vi "Autonomous Independent.vi"() -> ()   [LabVIEW 2017]
doc: "This VI is called when autonomous begins, and will automatically be terminated when autonomous ends. You can carry out timed or sensor driven robot movement independently without needing to return to the caller."
uses:
  <vilib>/Rock Robotics/WPI/ThirdParty/Phoenix-LabVIEW/Motor Controller/Controls/CTRE_Phoenix_MotorControl_ControlMode.ctl
  <vilib>/Rock Robotics/WPI/Utilities/WPI_GetSetVariantRefNum.vi
  <vilib>/Rock Robotics/Network Tables/NT Read String.vi
  <vilib>/Rock Robotics/Network Tables/NT Write Numeric Array.vi
  <vilib>/Rock Robotics/WPI/ThirdParty/Phoenix-LabVIEW/Motor Controller/Get/CTRE_Phoenix_MotorController_GetClosedLoopData.vi
  <vilib>/addons/control/pid/pid.llb/PID (DBL).vi
  <vilib>/Rock Robotics/WPI/RobotDrive/WPI_RobotDriveArcadeDrive_Standard(NoSaturation).vi
  <vilib>/addons/control/pid/NI_PID_pid.lvlib
panel:
  in  "PID gains 3":T1={"proportional gain (Kc)"=0.17, "integral time (Ti, min)"=0.002, "derivative time (Td, min)"=0.0}
  in  "setpoint 3":dbl format="%.2f"
  out "Yaw 3":dbl
  out "Closed-loop Error RF 14":i32
  out "Closed-loop Error LR 14":i32
  out "Closed-loop Error RF 13":i32
  out "Closed-loop Error LR 13":i32
  in  "PID gains 2":T1={"proportional gain (Kc)"=0.17, "integral time (Ti, min)"=0.002, "derivative time (Td, min)"=0.0}
  in  "setpoint 2":dbl format="%.2f"
  out "Yaw 2":dbl
  out "Closed-loop Error RF 12":i32
  out "Closed-loop Error LR 12":i32
  out "Closed-loop Error RF 11":i32
  out "Closed-loop Error LR 11":i32
  in  "Acceleration":i32=2100
  in  "Cruise Velocity":i32=1500
  out "Closed-loop Error LR":i32
  out "Closed-loop Error RF":i32
  in  "Lt Target 1":dbl=36500.0
  # "Be sure to right-click and choose Data Operations>>Make Current Value default if you want to save the array values with the VI"
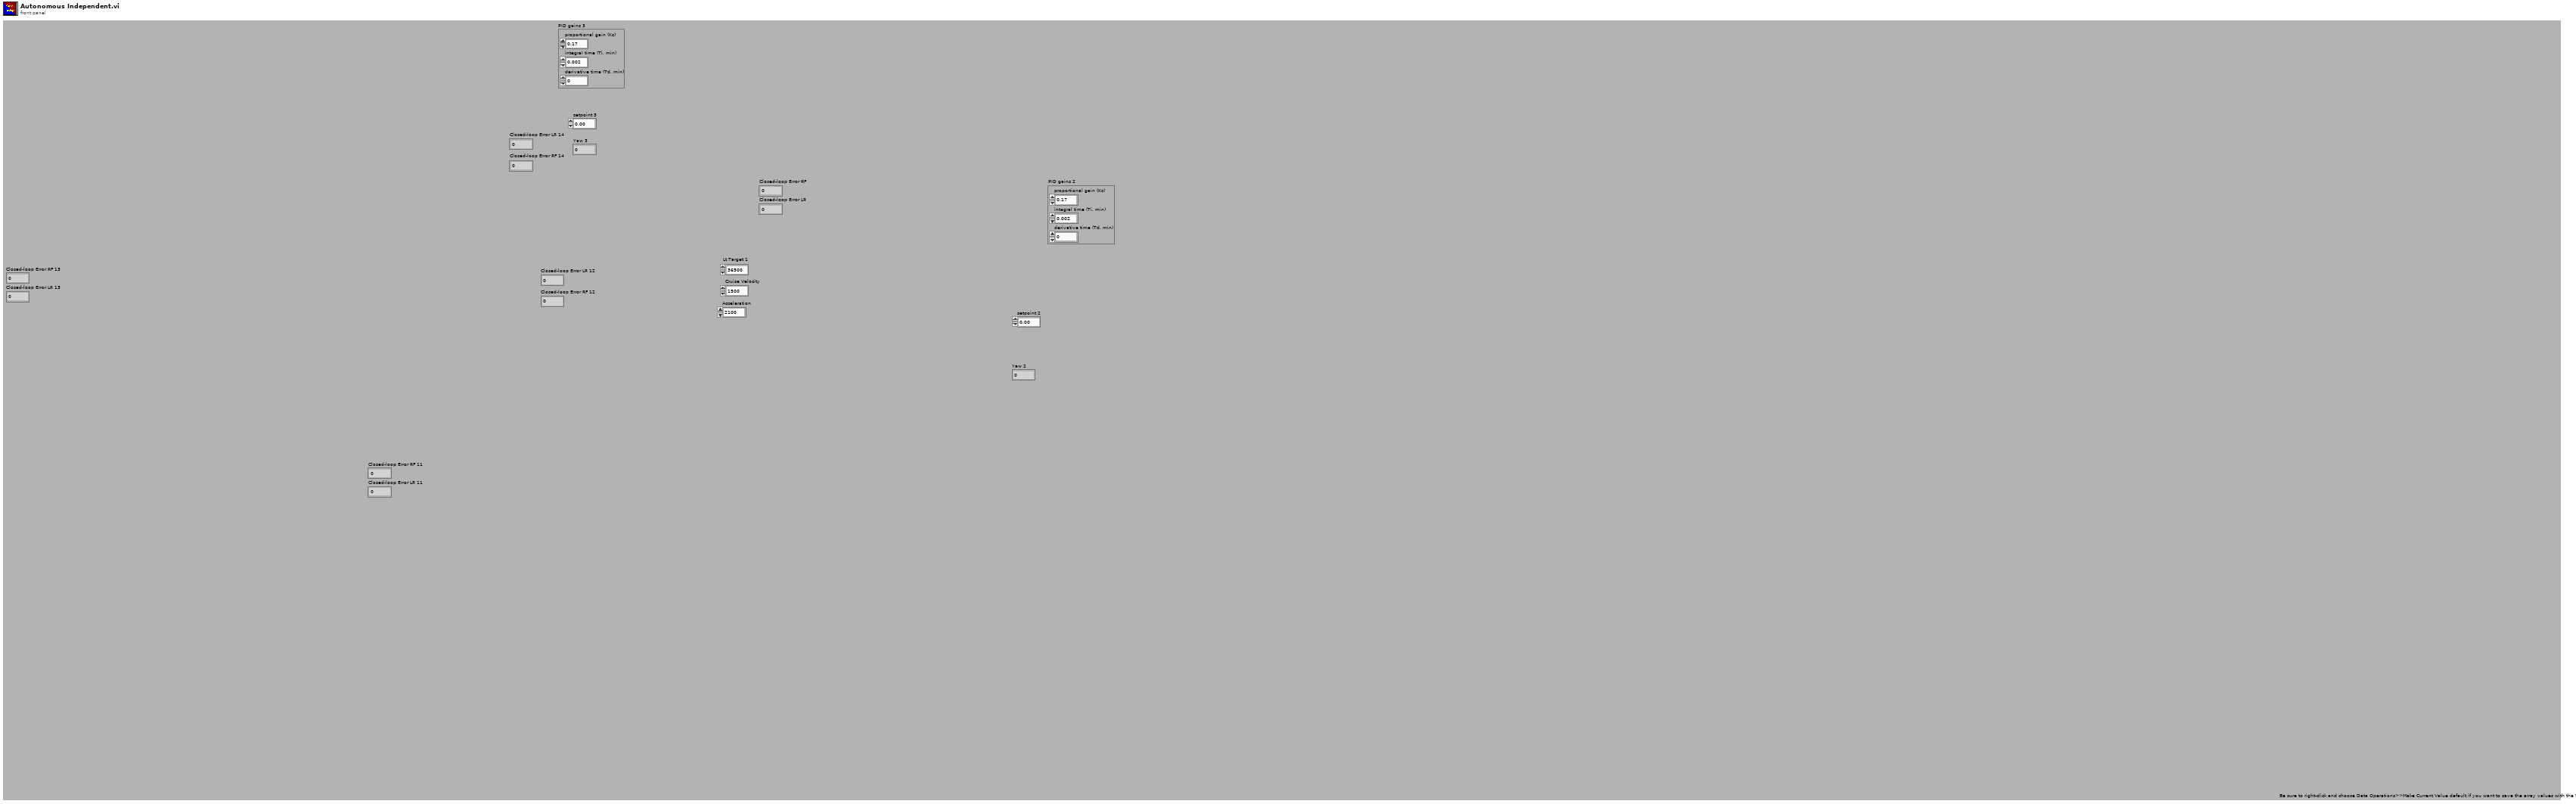
[diagram p1: front panel]
types:
  T1 = cluster{"proportional gain (Kc)":dbl, "integral time (Ti, min)":dbl, "derivative time (Td, min)":dbl}
  T2 = typedef "WPI_MotorControlDeviceRef.ctl" = cluster{"DeviceStatus":errorcluster, "Type":T3, "PWM":cluster{"PWM Channel":T4, "DeadBand":T5}, "CAN":cluster{"Device Number":u8, "SetOutput VI Ref":variant, "GetOutput VI Ref":variant, "Enable VI Ref":variant, "Disable VI Ref":variant, "Data":variant}, "Invert":bool, "DIO PWM":cluster{"PWM \"Enable\" Channel":T4, "DIOChannel":T6, "PWM Rate":dbl}}
  T3 = typedef "WPI_MotorControlType.ctl" = enum16{"PWM", "CAN", "DIO PWM"}
  T4 = typedef "FPGA_DIOPWMChannel.ctl" = enum8{"PWM 0", "PWM 1", "PWM 2", "PWM 3", "PWM 4", "PWM 5", "PWM 6", "PWM 7", "PWM 8", "PWM 9", "PWM MXP 0", "PWM MXP 1", "PWM MXP 2", "PWM MXP 3", "PWM MXP 4", "PWM MXP 5", "PWM MXP 6", "PWM MXP 7", "PWM MXP 8", "PWM MXP 9", "Invalid"}
  T5 = typedef "WPI_PWMDeadband.ctl" = cluster{"Name":string, "maxPositivePwm":i32, "minPositivePwm":i32, "centerPwm":i32, "maxNegativePwm":i32, "minNegativePwm":i32, "angularRange":u16}
  T6 = typedef "FPGA_DIOChannel.ctl" = enum8{"DIO 0", "DIO 1", "DIO 2", "DIO 3", "DIO 4", "DIO 5", "DIO 6", "DIO 7", "DIO 8", "DIO 9", "DIO MXP 0", "DIO MXP 1", "DIO MXP 2", "DIO MXP 3", "DIO MXP 4", "DIO MXP 5", "DIO MXP 6", "DIO MXP 7", "DIO MXP 8", "DIO MXP 9", "DIO MXP 10", "DIO MXP 11", "DIO MXP 12", "DIO MXP 13", "DIO MXP 14", "DIO MXP 15", "SPI Port CS1", "SPI Port CS2", "SPI Port CS3", "SPI Port MISO", "SPI Port MOSI", "Invalid"}
  T7 = typedef "WPI_JoystickDevRef.ctl" = cluster{"Device":T8}
  T8 = typedef "WPI_JoystickDeviceEnum.ctl" = enum16{"USB 0", "USB 1", "USB 2", "USB 3", "USB 4", "USB 5"}
  T9 = typedef "CTRE_Phoenix_MotorControl_ControlMode.ctl" = u16
  T10 = cluster{"Yaw":dbl, "Roll":dbl, "Pitch":dbl, "Heading":dbl, "Fused Heading":dbl}
  T11 = typedef "WPI_RobotDriveDevRef.ctl" = cluster{"DevStatus":errorcluster, "Motors[]":T2[], "Square Inputs":bool, "Max Output":dbl}
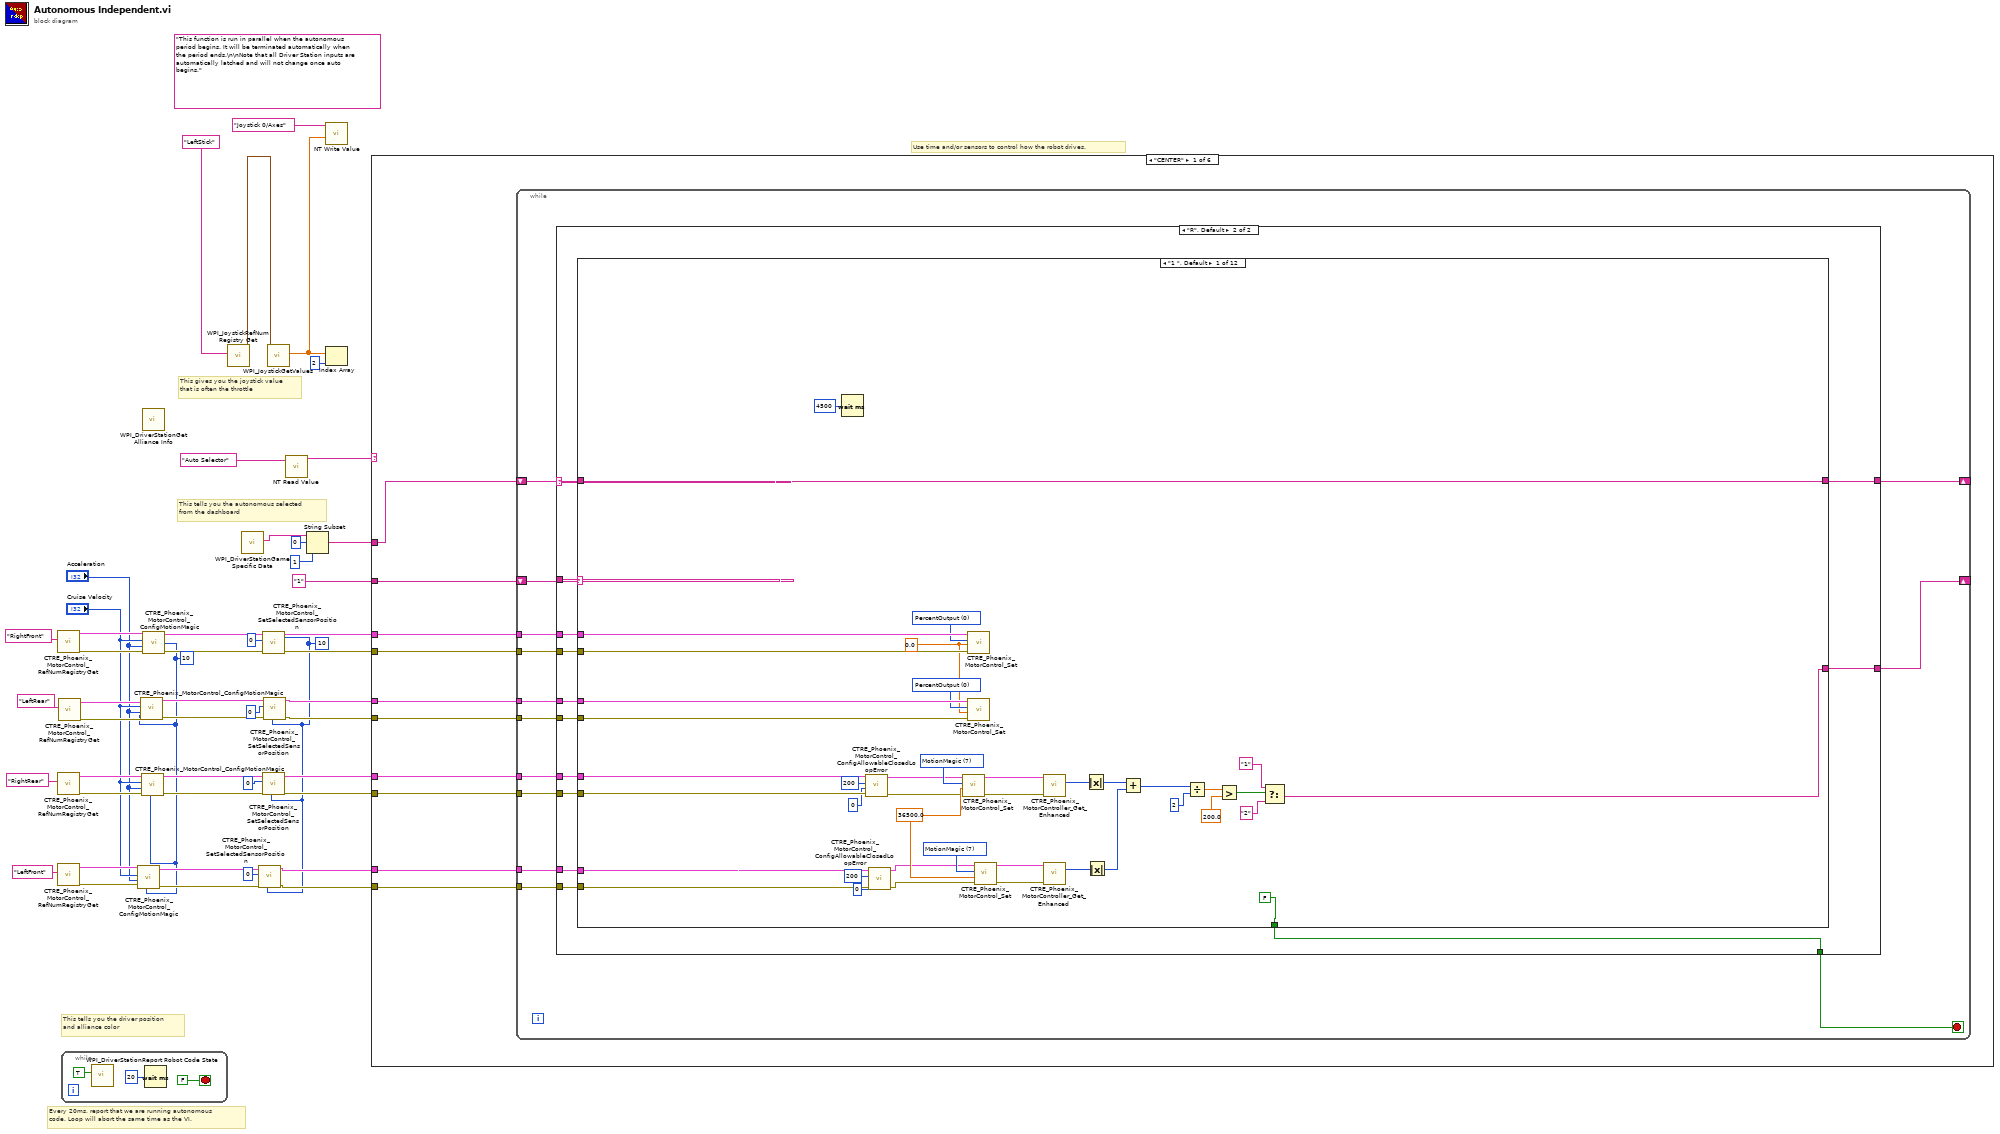
[diagram p0: block diagram]
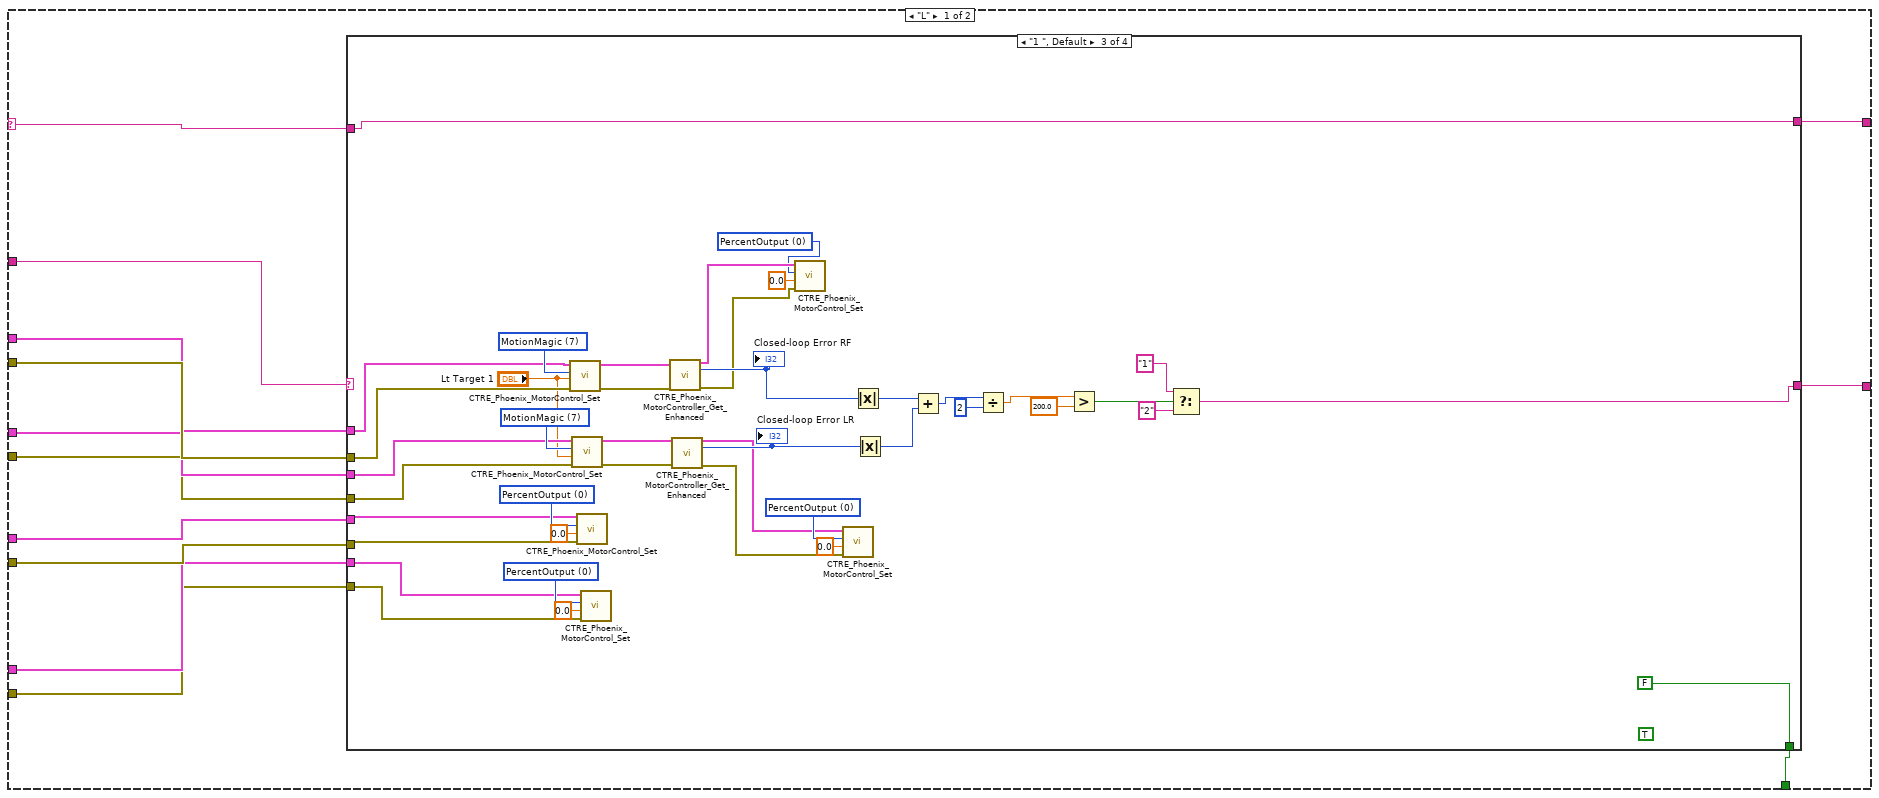
[diagram p2: hidden frame]
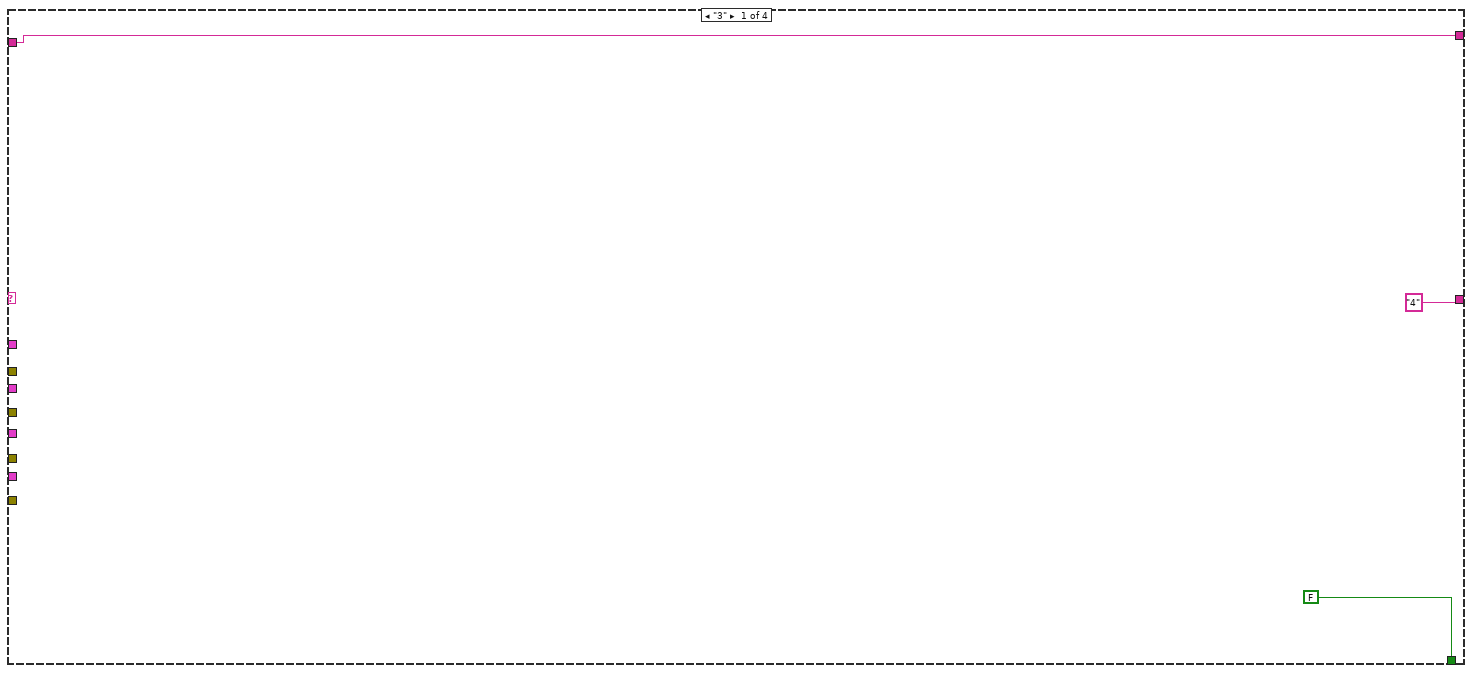
[diagram p3: hidden frame]
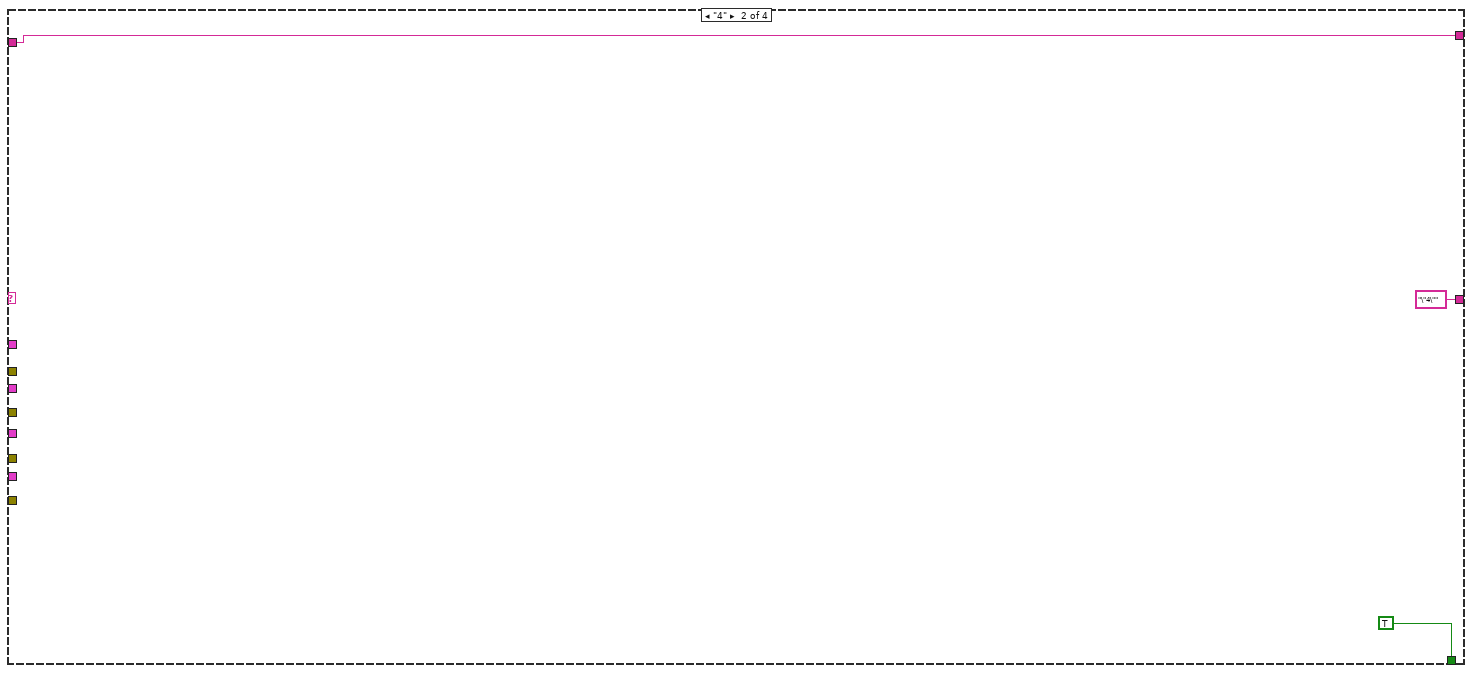
[diagram p4: hidden frame]
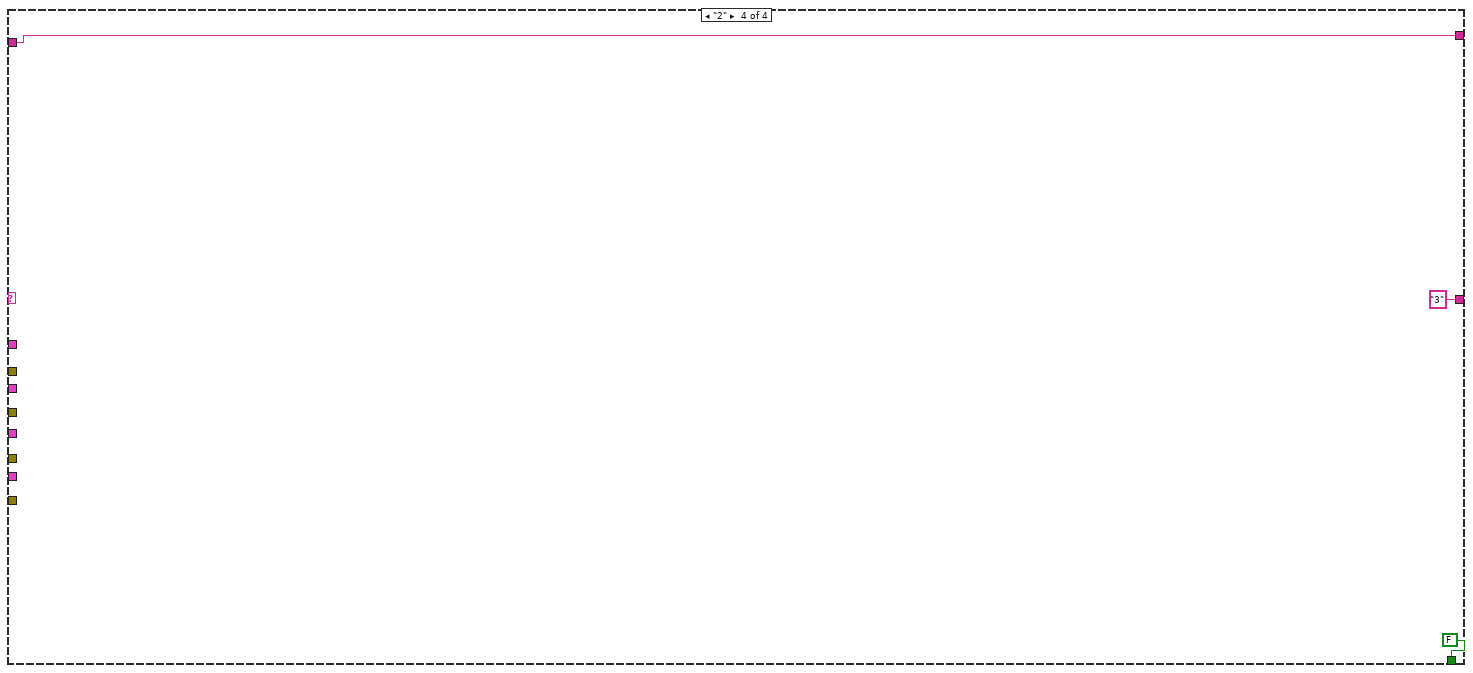
[diagram p5: hidden frame]
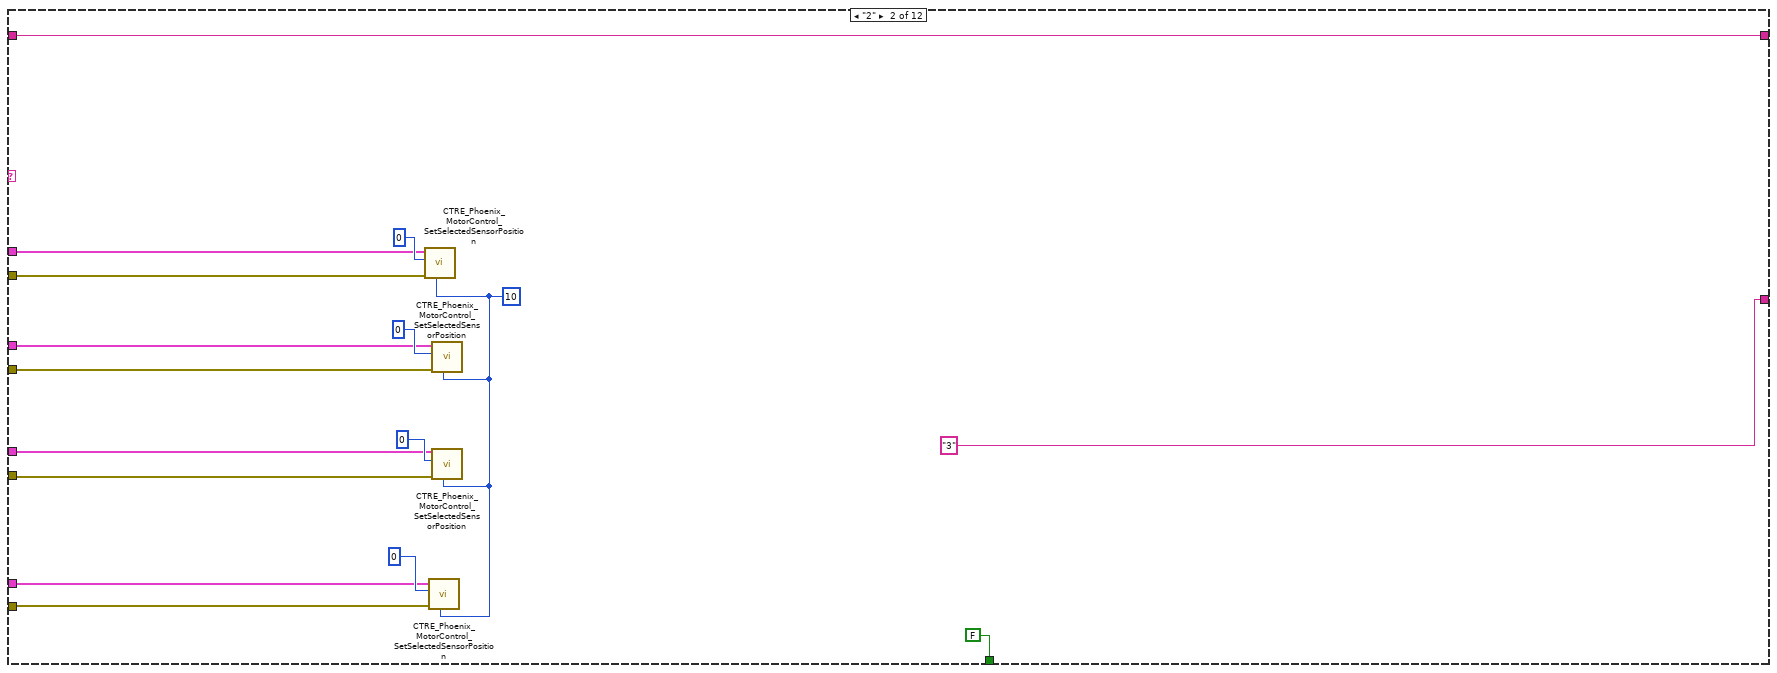
[diagram p6: hidden frame]
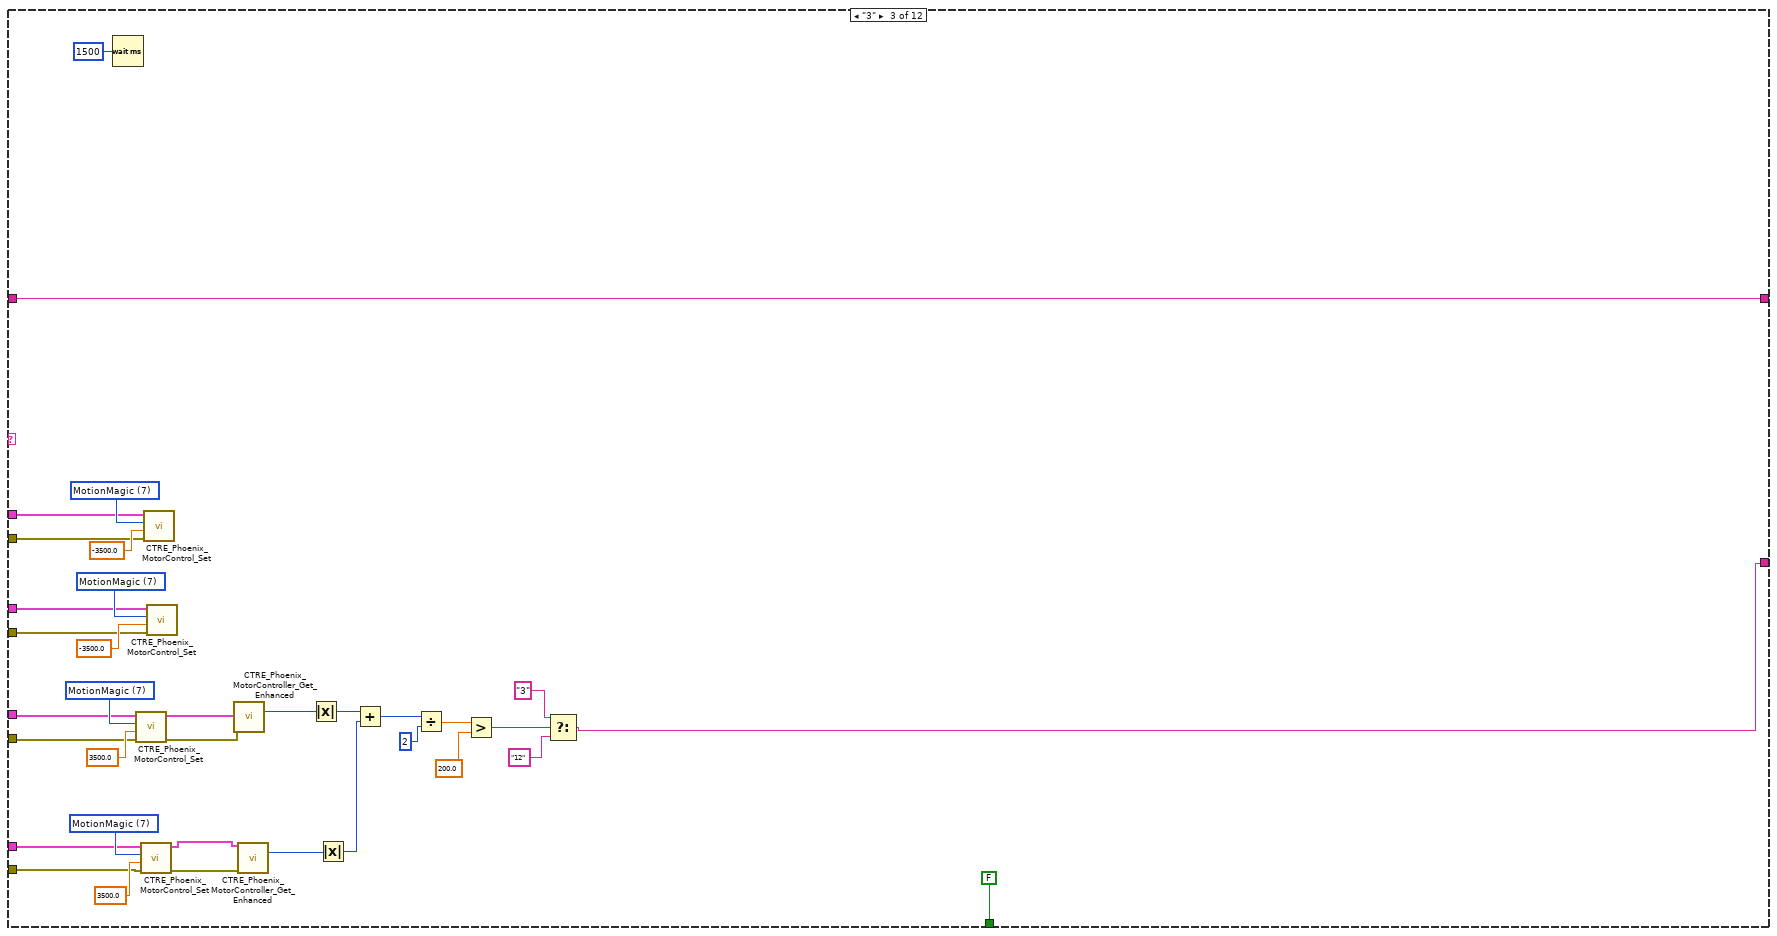
[diagram p7: hidden frame]
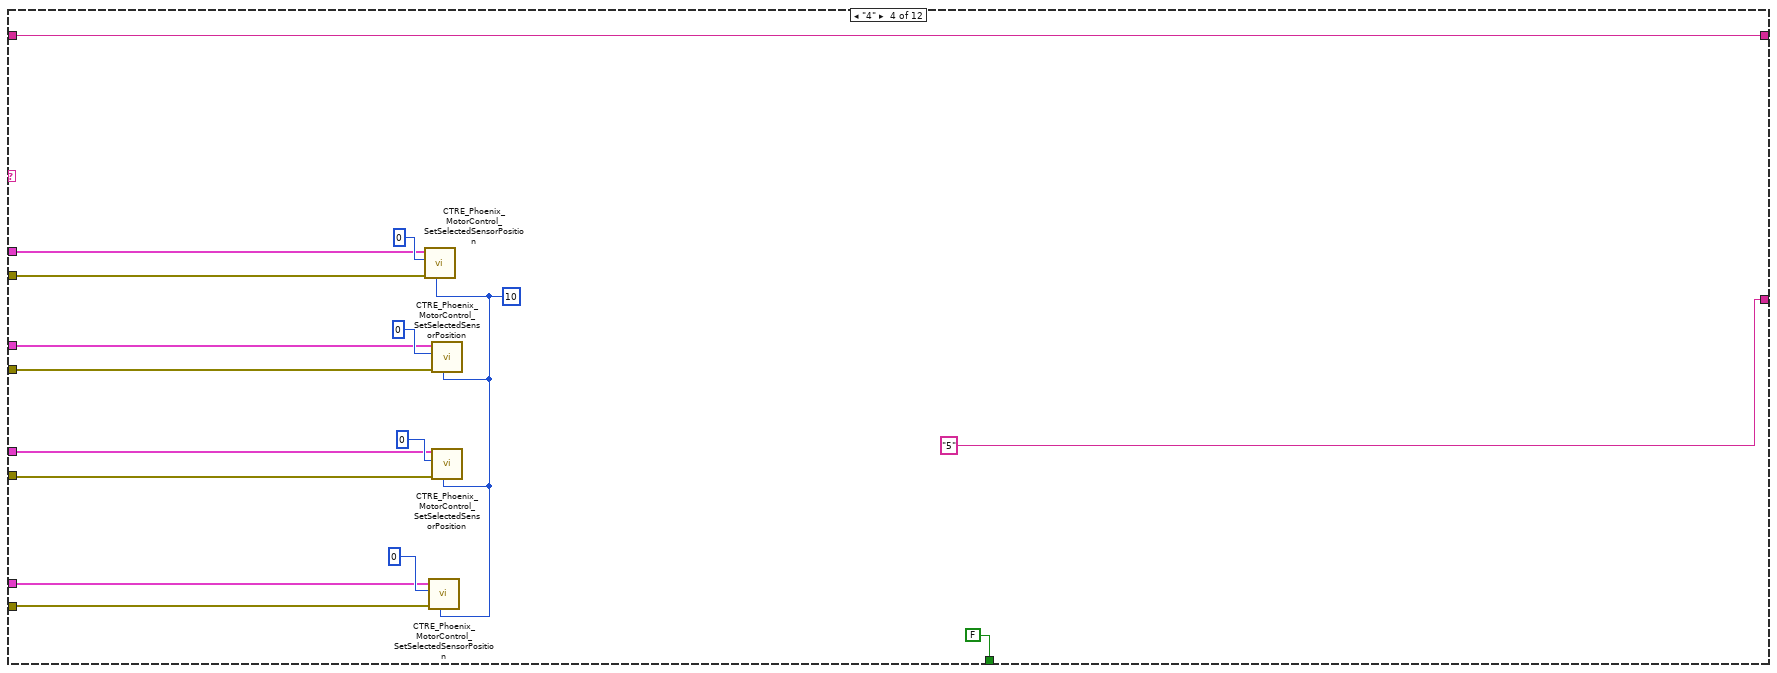
[diagram p8: hidden frame]
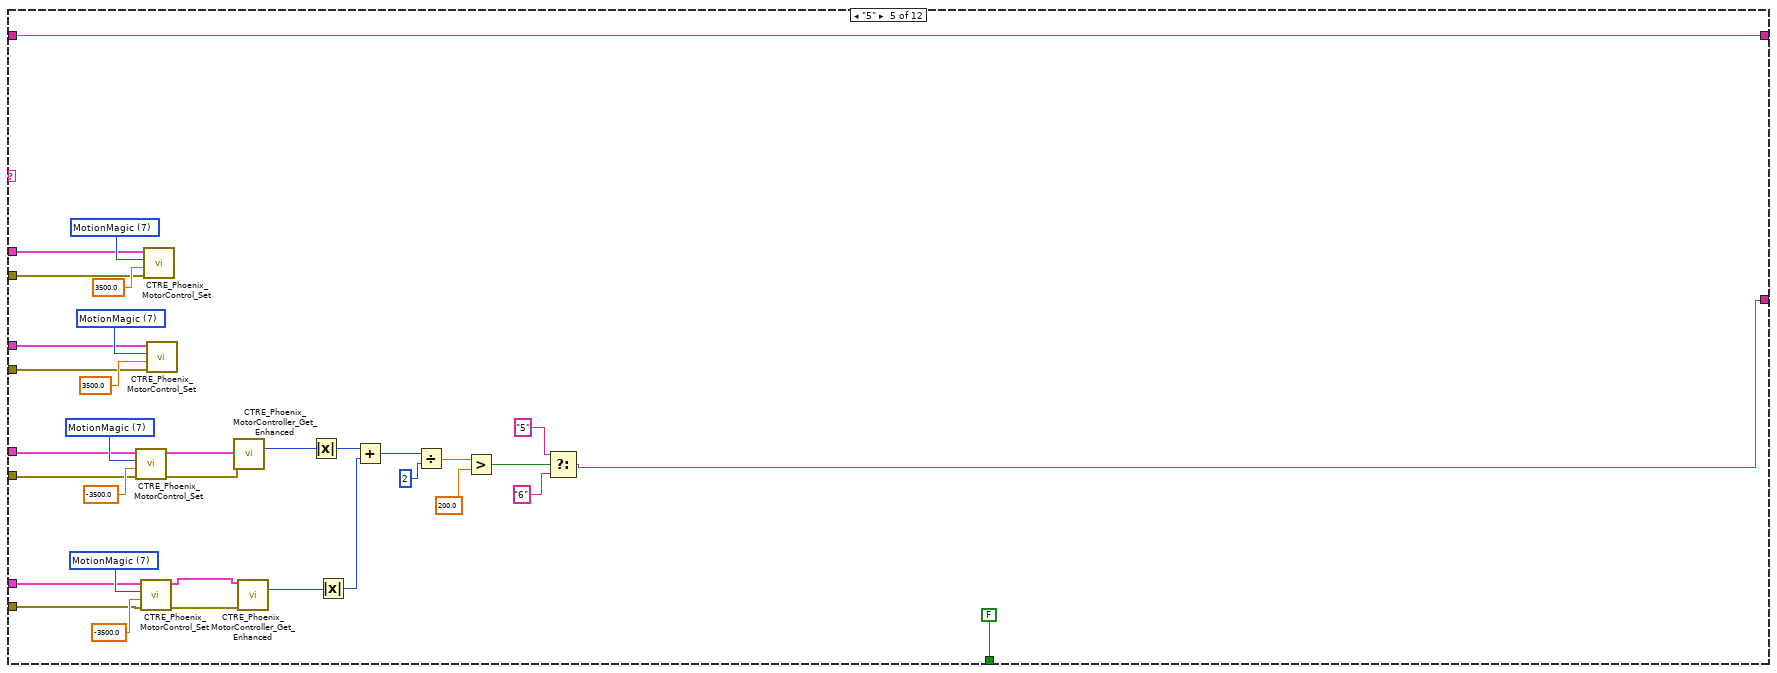
[diagram p9: hidden frame]
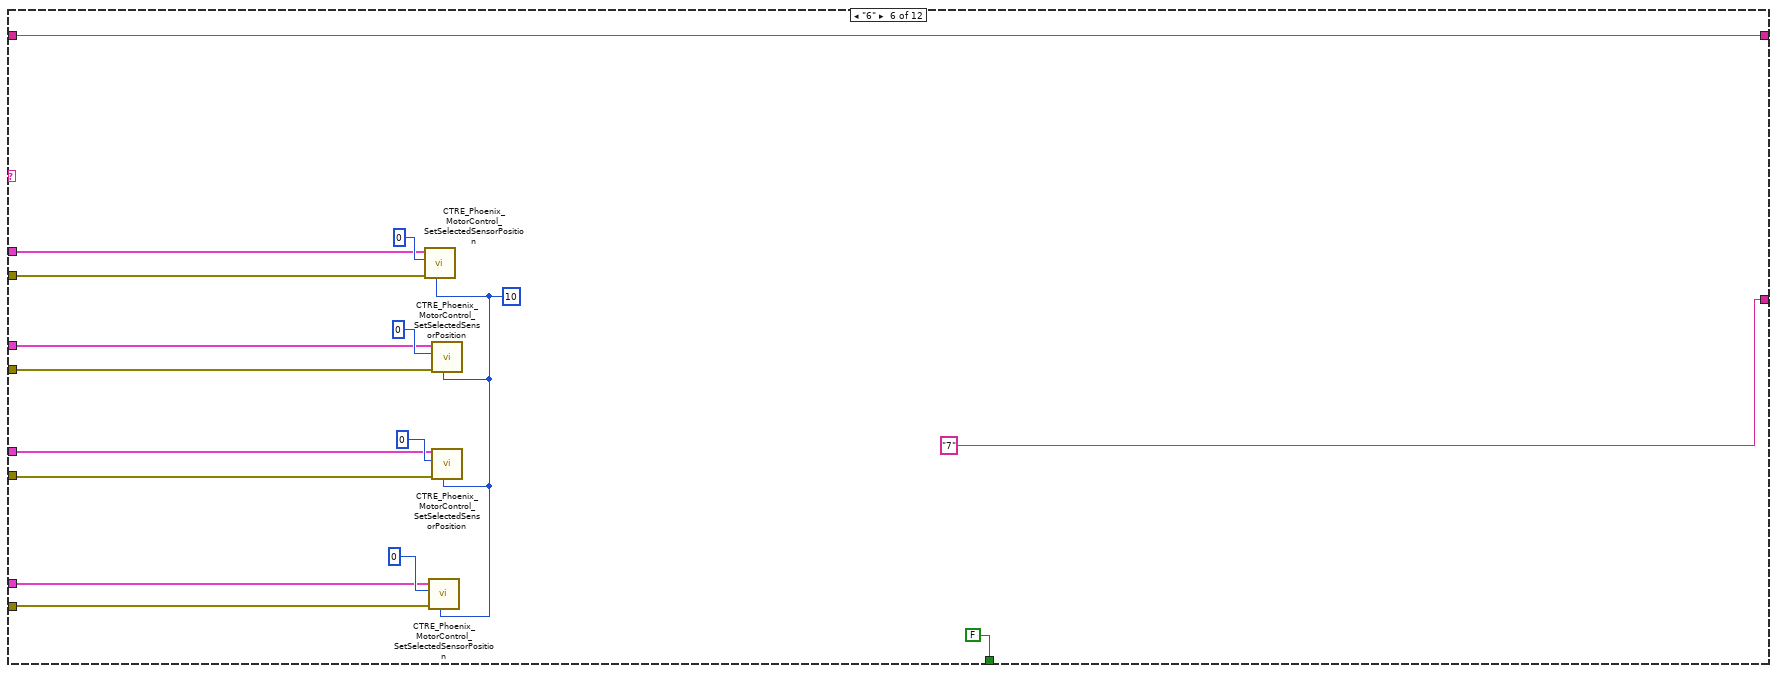
[diagram p10: hidden frame]
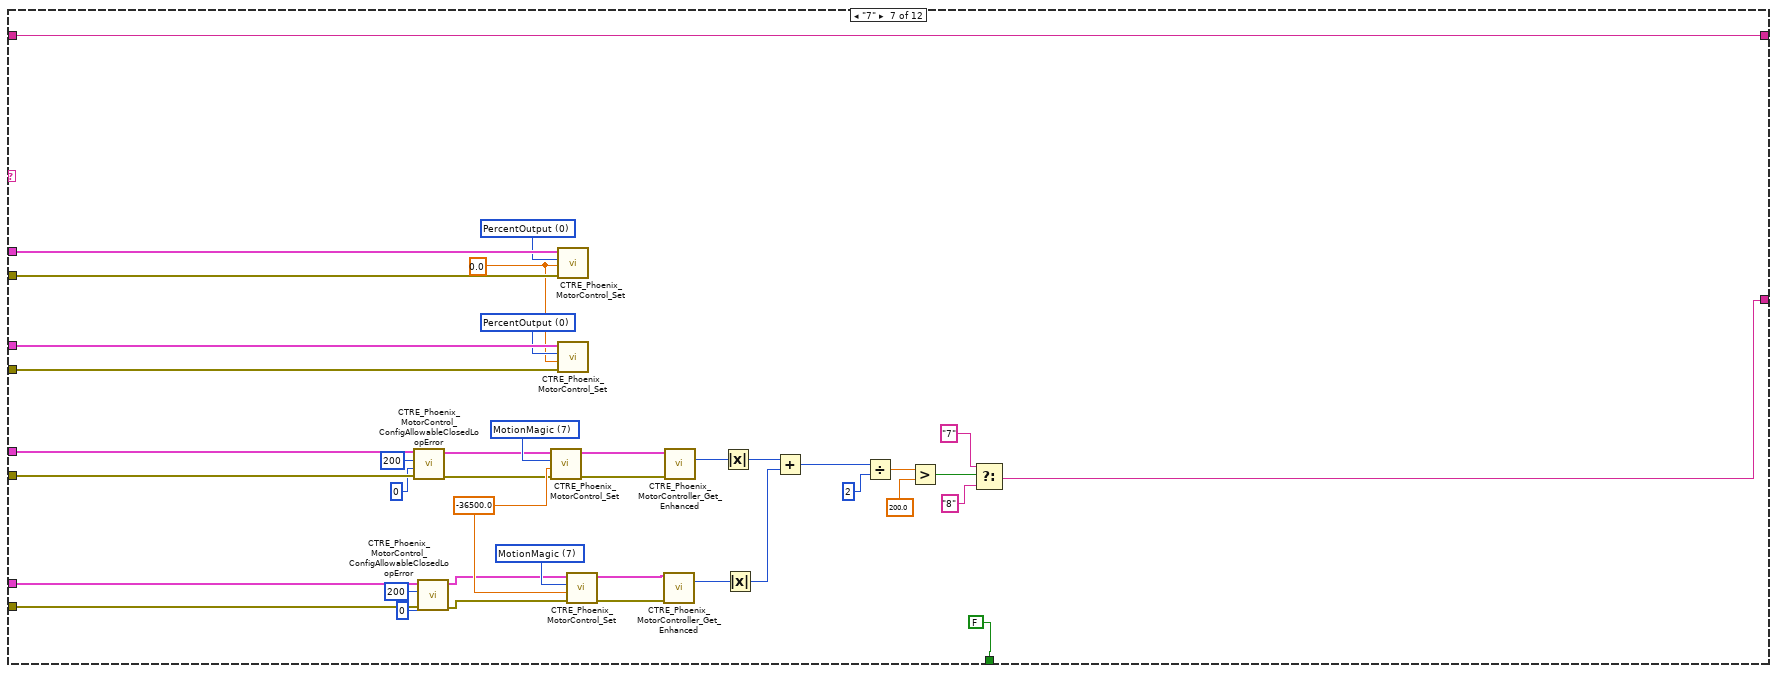
[diagram p11: hidden frame]
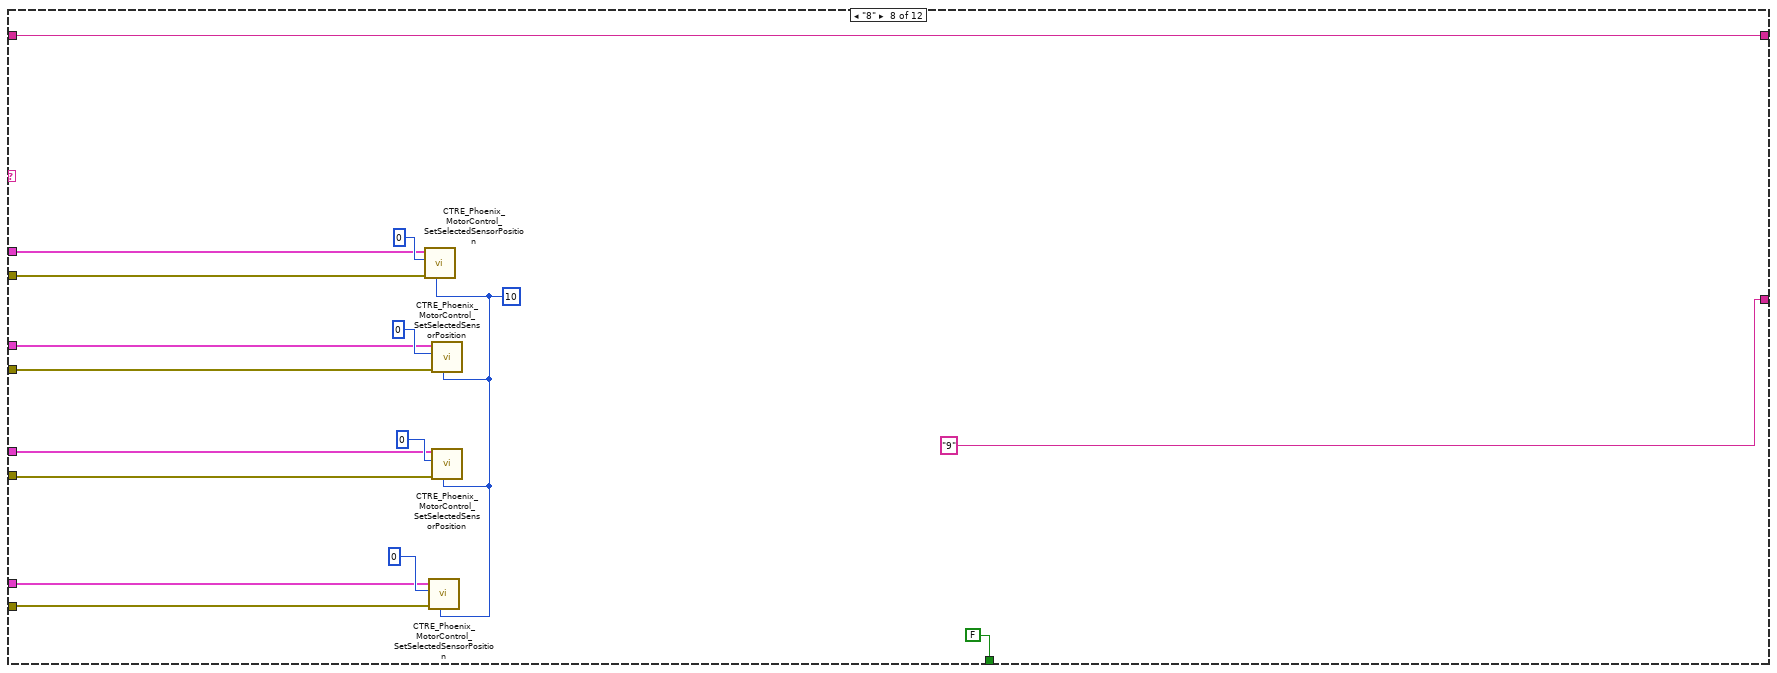
[diagram p12: hidden frame]
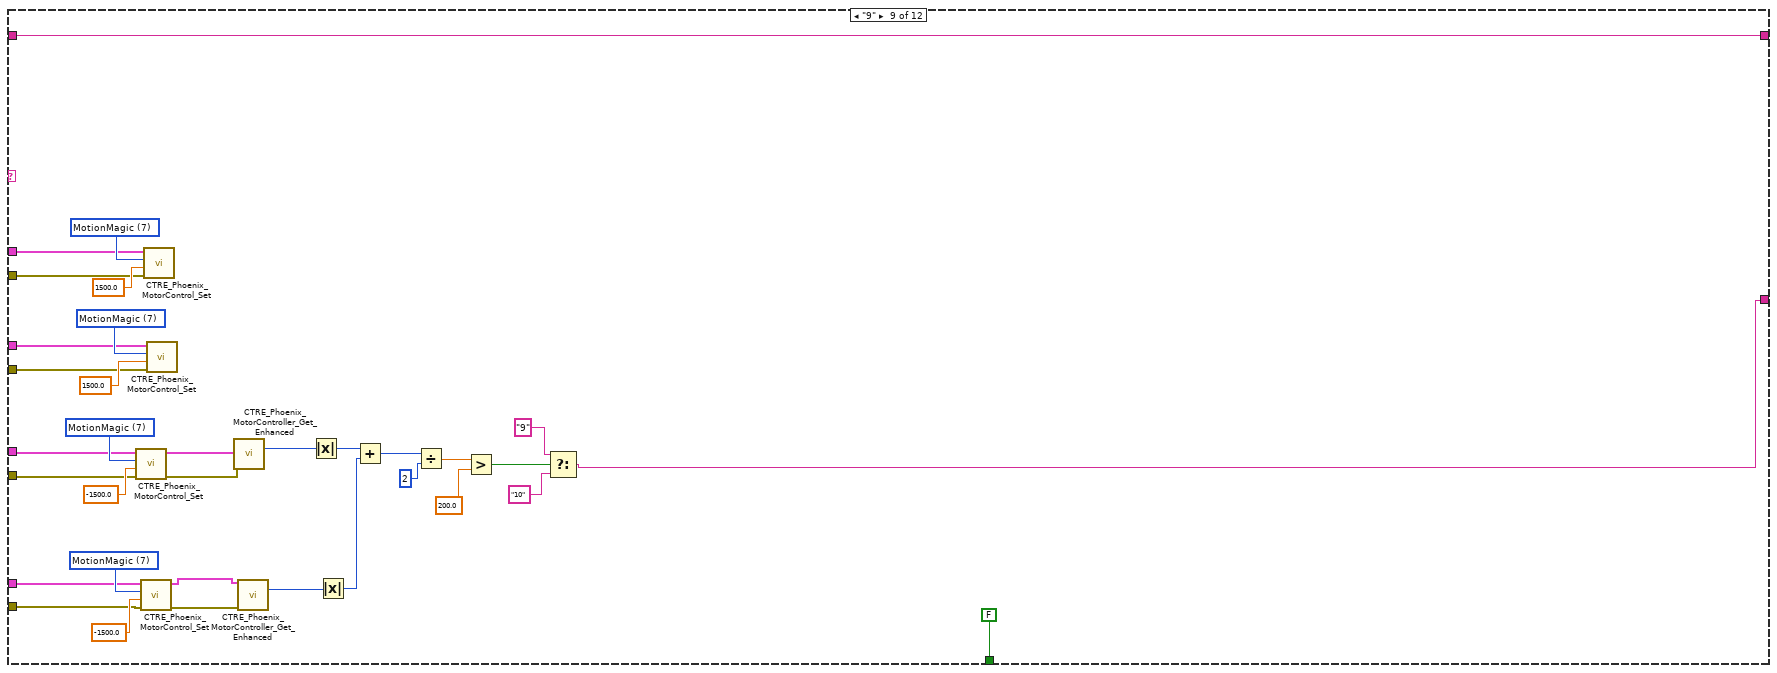
[diagram p13: hidden frame]
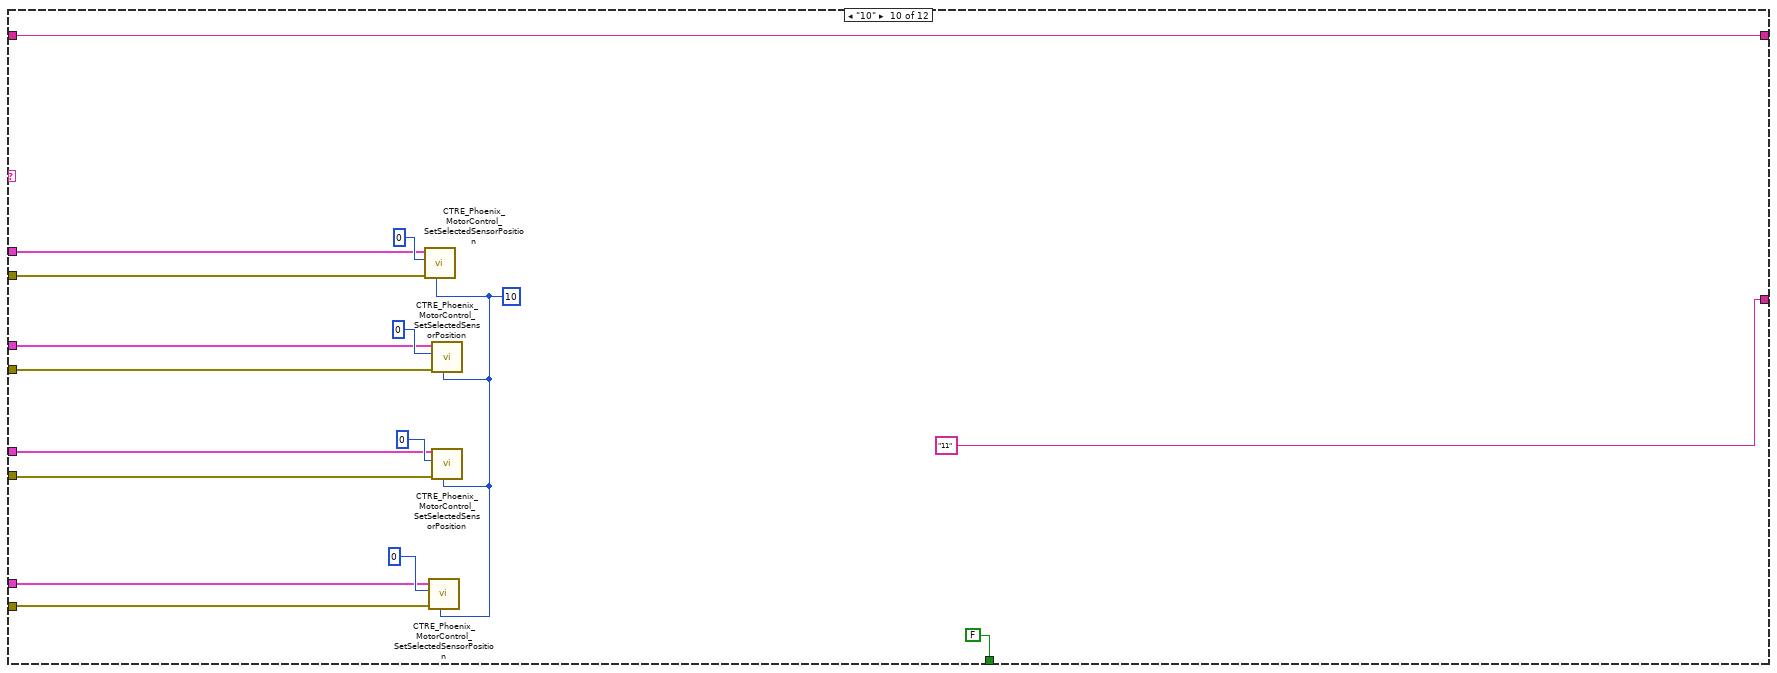
[diagram p14: hidden frame]
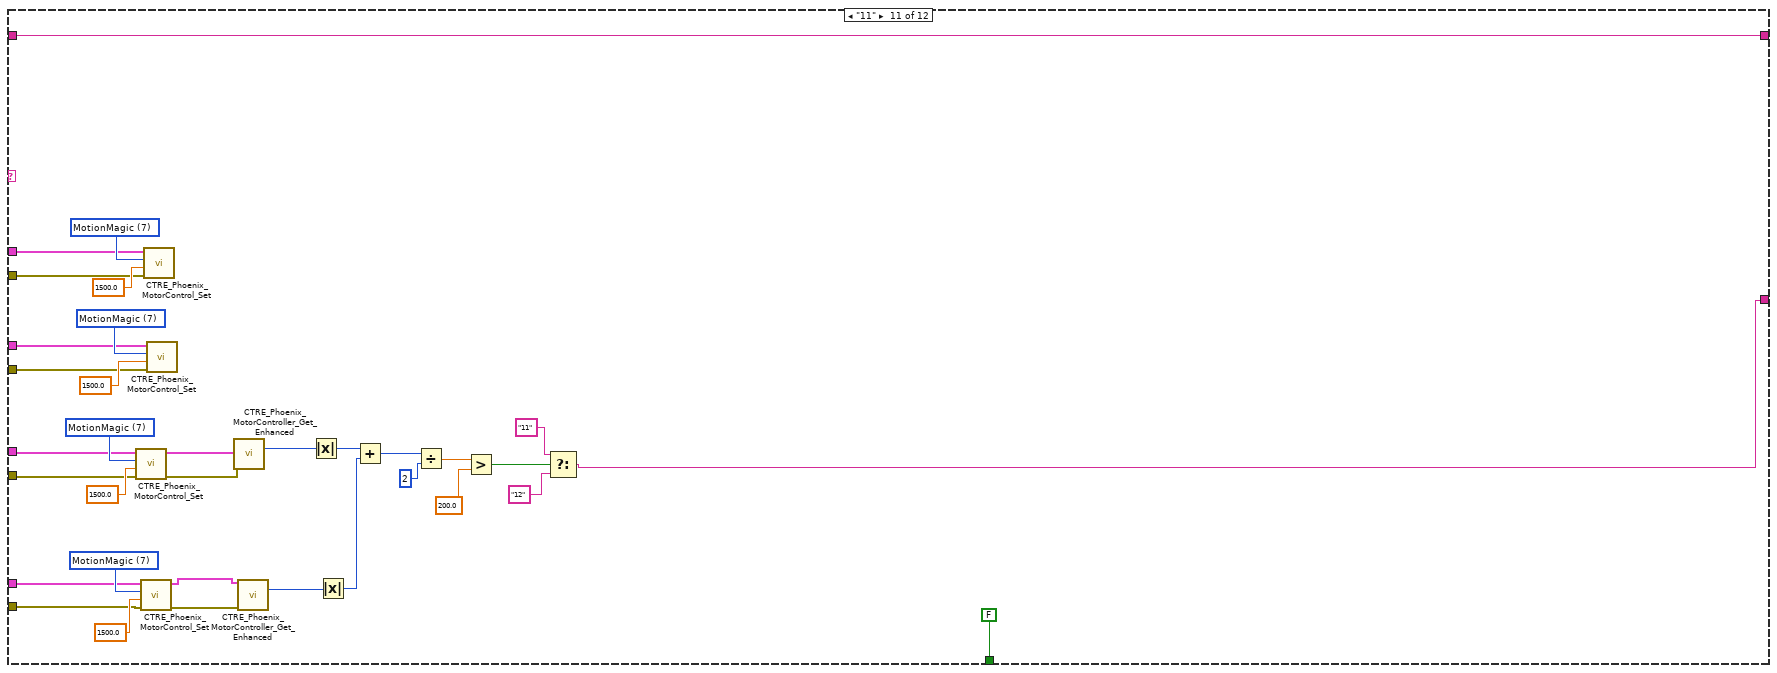
[diagram p15: hidden frame]
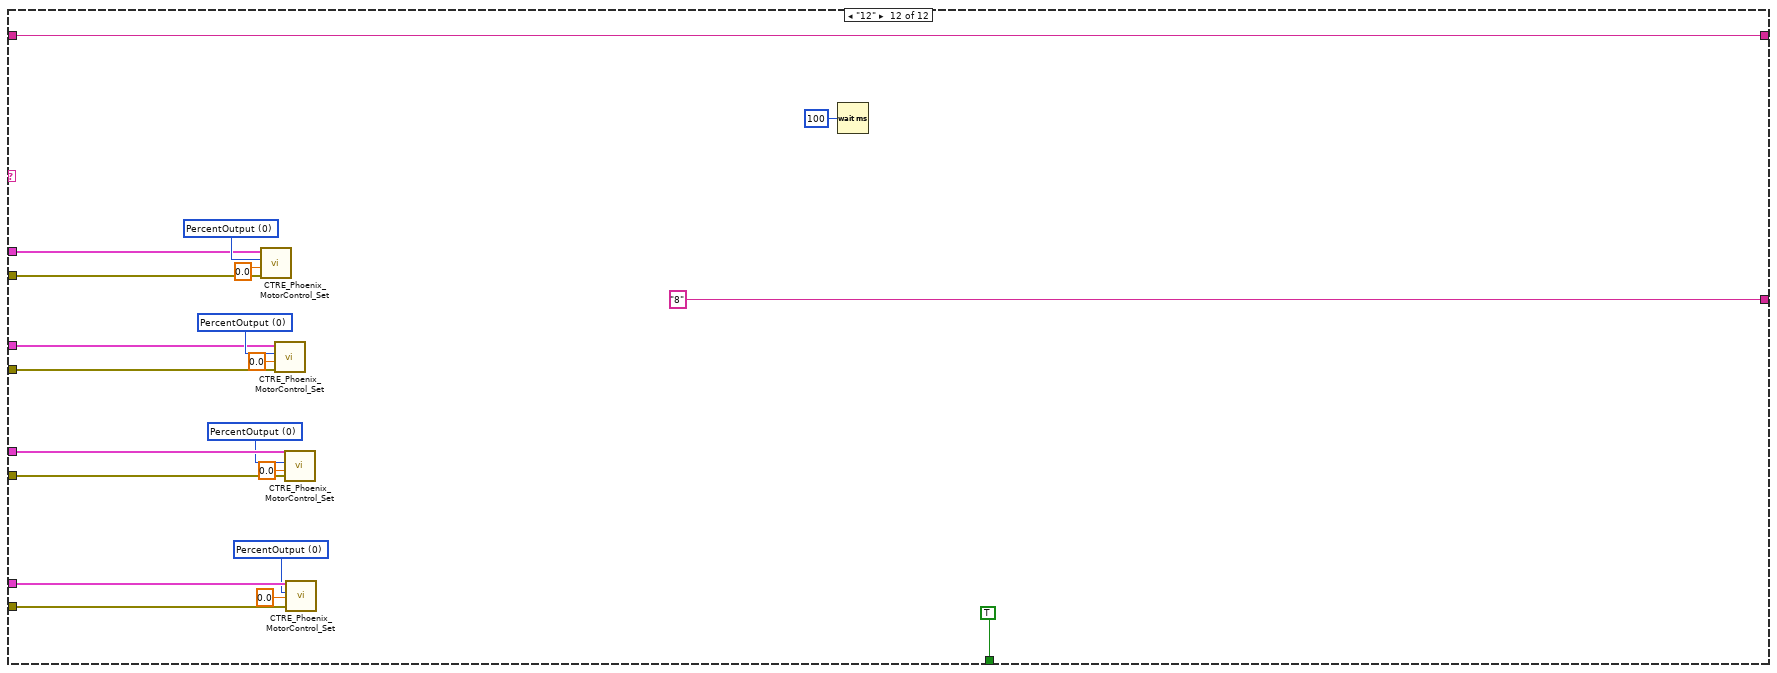
[diagram p16: hidden frame]
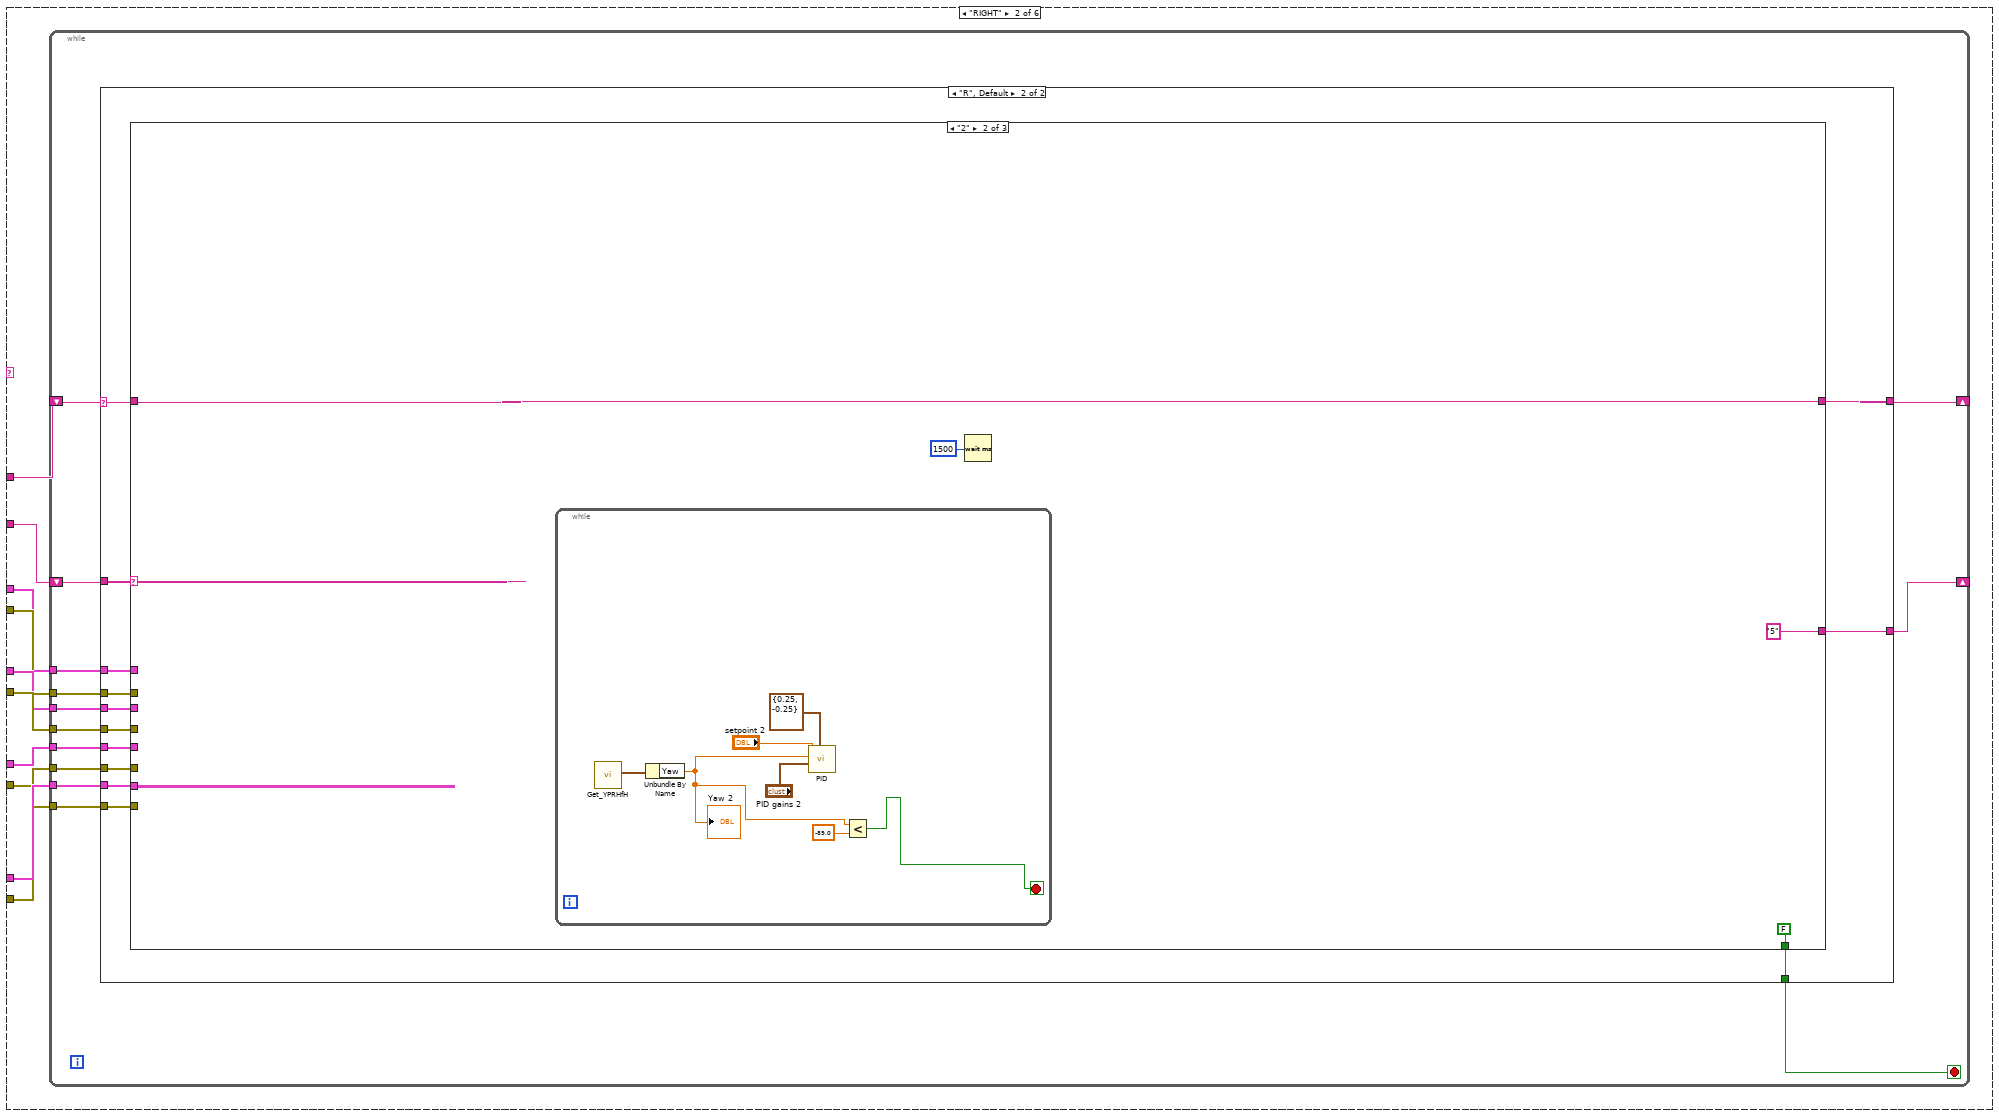
[diagram p17: hidden frame]
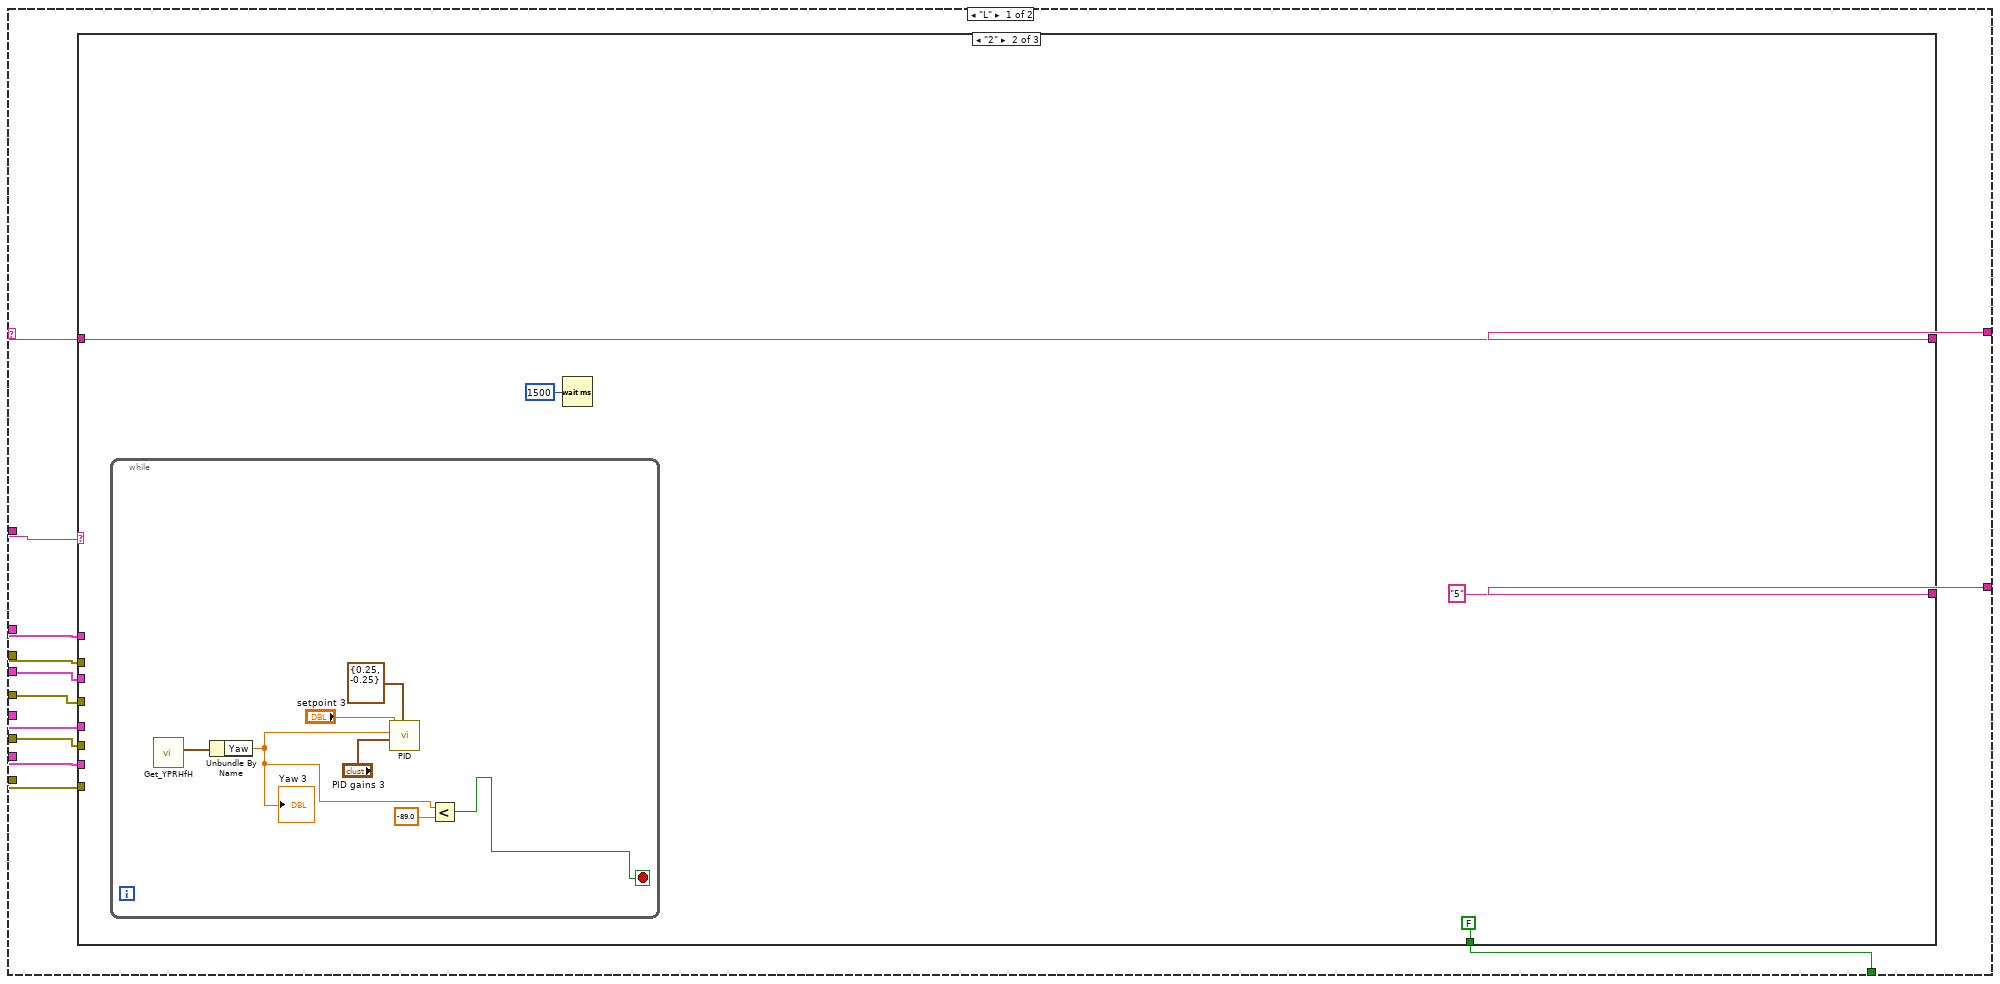
[diagram p18: hidden frame]
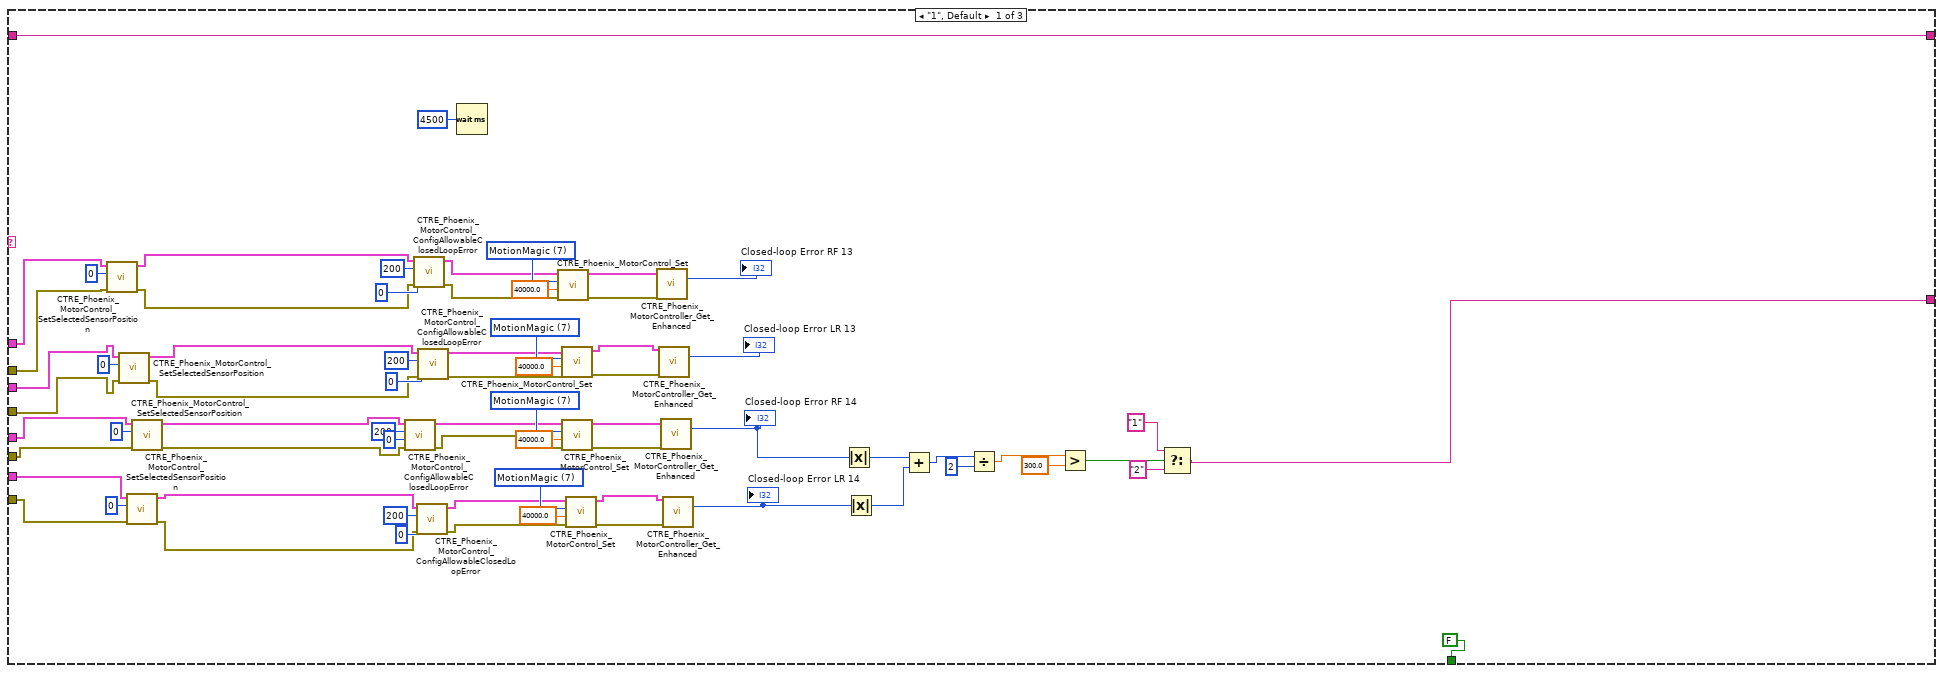
[diagram p19: hidden frame]
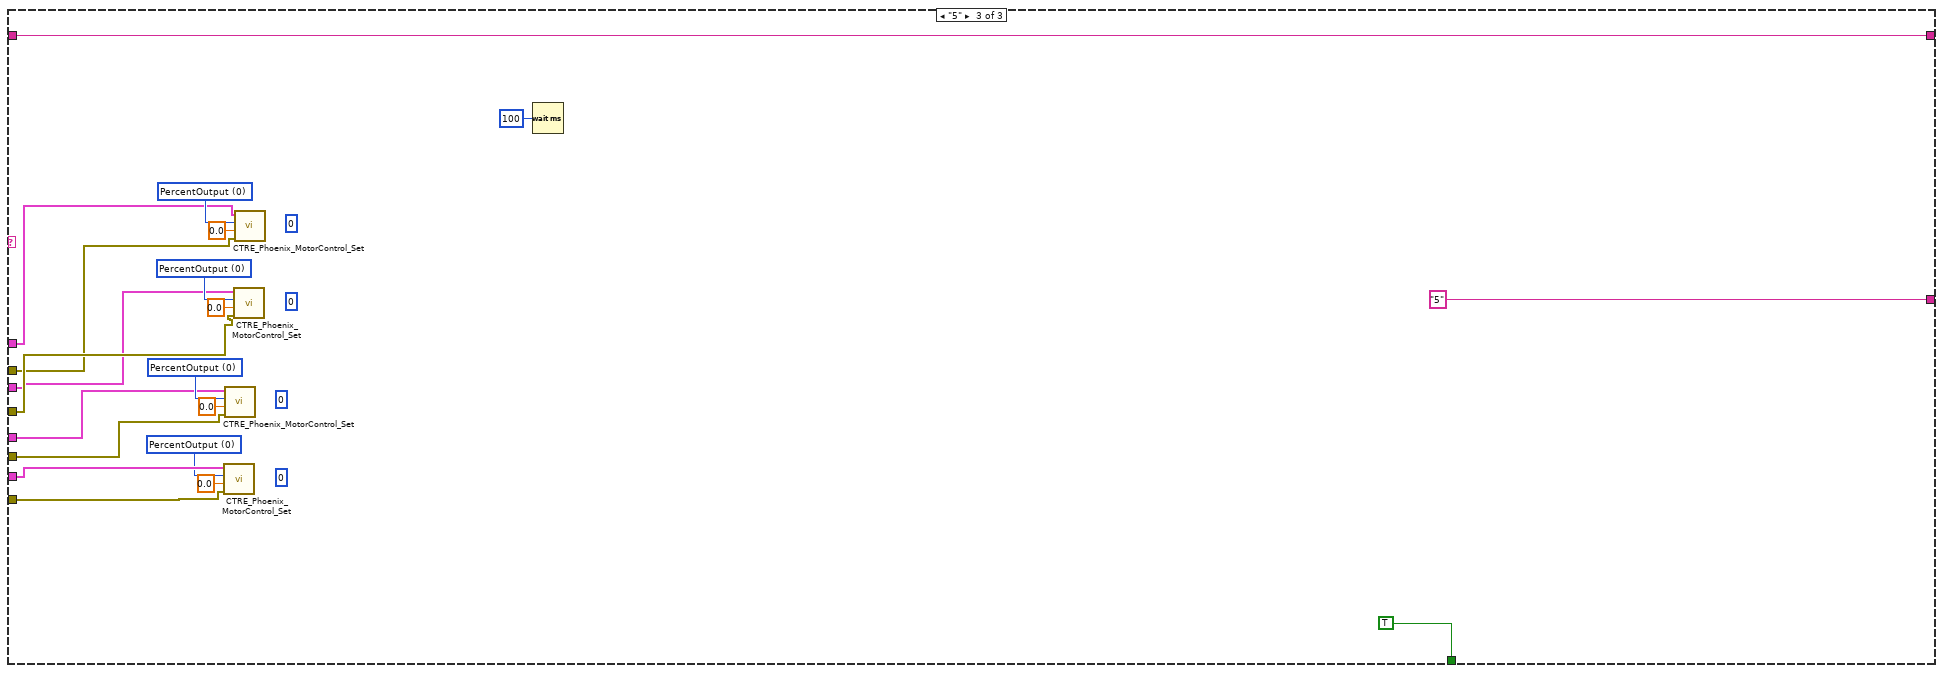
[diagram p20: hidden frame]
diagram:
  w2 = u32 10 ("timeoutMs")
  w1 = u32 10 ("timeoutMs")
  (unwired) "This function is run in parallel when the autonomous period begins. It will be terminated automatically when the period ends.\n\nNote that all Driver Station inputs are automatically latched and will not change once auto begins."
  # "This tells you the autonomous selected\nfrom the dashboard"
  # "Every 20ms, report that we are running autonomous\ncode. Loop will abort the same time as the VI."
  # "This gives you the joystick value\nthat is often the throttle"
  # "Use time and/or sensors to control how the robot drives."
  # "This tells you the driver position\nand alliance color"
  n1 = call <vilib>:"CTRE_Phoenix_MotorControl_RefNumRegistryGet.vi"("refnum name"="RightFront") -> ("error out"=w20:errorcluster, "PhoenixMotorControlDevRef"=w21:T2)  [unwired: 9 in]
  n2 = call <vilib>:"CTRE_Phoenix_MotorControl_RefNumRegistryGet.vi"("refnum name"="RightRear") -> ("error out"=w16:errorcluster, "PhoenixMotorControlDevRef"=w17:T2)  [unwired: 9 in]
  n3 = call <vilib>:"CTRE_Phoenix_MotorControl_RefNumRegistryGet.vi"("refnum name"="LeftFront") -> ("error out"=w14:errorcluster, "PhoenixMotorControlDevRef"=w15:T2)  [unwired: 9 in]
  n4 = call <vilib>:"CTRE_Phoenix_MotorControl_RefNumRegistryGet.vi"("refnum name"="LeftRear") -> ("error out"=w18:errorcluster, "PhoenixMotorControlDevRef"=w19:T2)  [unwired: 9 in]
  n5 = while {
    stop <- FALSE stop-if-true
    n6 = call <vilib>:"WPI_DriverStationReport Robot Code State.vi"("Autonomous"=TRUE) -> ()  [unwired: 10 in, 1 out]
    n7 = Wait (ms)(milliseconds to wait=u32 20) -> ()  [unwired: 1 out]
  }
  n8 = call <vilib>:"CTRE_Phoenix_MotorControl_ConfigMotionMagic.vi"("timeoutMs"=w2, "error in (no error)"=w14, "Acceleration"="Acceleration", "Cruise Velocity"="Cruise Velocity", "PhoenixMotorControlDevRef"=w15) -> ("error out"=w6:errorcluster, "PhoenixMotorControlDevRef"=w7:T2)  [unwired: 5 in]
  n9 = call <vilib>:"CTRE_Phoenix_MotorControl_ConfigMotionMagic.vi"("timeoutMs"=w2, "error in (no error)"=w18, "Acceleration"="Acceleration", "Cruise Velocity"="Cruise Velocity", "PhoenixMotorControlDevRef"=w19) -> ("error out"=w10:errorcluster, "PhoenixMotorControlDevRef"=w11:T2)  [unwired: 5 in]
  n10 = call <vilib>:"CTRE_Phoenix_MotorControl_ConfigMotionMagic.vi"("timeoutMs"=w2, "error in (no error)"=w16, "Acceleration"="Acceleration", "Cruise Velocity"="Cruise Velocity", "PhoenixMotorControlDevRef"=w17) -> ("error out"=w8:errorcluster, "PhoenixMotorControlDevRef"=w9:T2)  [unwired: 5 in]
  n11 = call <vilib>:"WPI_DriverStationGet Alliance Info.vi"() -> ()  [unwired: 12 out]
  n12 = call <vilib>:"CTRE_Phoenix_MotorControl_ConfigMotionMagic.vi"("timeoutMs"=w2, "error in (no error)"=w20, "Acceleration"="Acceleration", "Cruise Velocity"="Cruise Velocity", "PhoenixMotorControlDevRef"=w21) -> ("error out"=w12:errorcluster, "PhoenixMotorControlDevRef"=w13:T2)  [unwired: 5 in]
  n13 = call <vilib>:"WPI_JoystickRefNum Registry Get.vi"("refnum name"="LeftStick") -> ("JoystickDevRef"=w47:T7)  [unwired: 1 in, 9 out]
  n14 = call <vilib>:"WPI_DriverStationGame Specific Data.vi"() -> ("Game Specific Data"=w41:string)  [unwired: 11 in]
  n15 = call <vilib>:"CTRE_Phoenix_MotorControl_SetSelectedSensorPosition.vi"("timeoutMs"=w1, "error in (no error)"=w6, "New Sensor Position"=0, "PhoenixMotorControlDevRef"=w7) -> ("error out"=w24:errorcluster, "PhoenixMotorControlDevRef"=w25:T2)  [unwired: 6 in]
  n16 = call <vilib>:"CTRE_Phoenix_MotorControl_SetSelectedSensorPosition.vi"("timeoutMs"=w1, "error in (no error)"=w12, "New Sensor Position"=0, "PhoenixMotorControlDevRef"=w13) -> ("error out"=w31:errorcluster, "PhoenixMotorControlDevRef"=w3:T2)  [unwired: 6 in]
  n17 = call <vilib>:"CTRE_Phoenix_MotorControl_SetSelectedSensorPosition.vi"("timeoutMs"=w1, "error in (no error)"=w8, "New Sensor Position"=0, "PhoenixMotorControlDevRef"=w9) -> ("error out"=w26:errorcluster, "PhoenixMotorControlDevRef"=w27:T2)  [unwired: 6 in]
  n18 = call <vilib>:"CTRE_Phoenix_MotorControl_SetSelectedSensorPosition.vi"("timeoutMs"=w1, "error in (no error)"=w10, "New Sensor Position"=0, "PhoenixMotorControlDevRef"=w11) -> ("error out"=w28:errorcluster, "PhoenixMotorControlDevRef"=w29:T2)  [unwired: 6 in]
  n19 = call <vilib>:"WPI_JoystickGetValues.vi"("JoystickDevRef"=w47) -> ("Axes"=w43:dbl[])  [unwired: 6 in, 4 out]
  n20 = call-poly <vilib>:"NT Read Value.vi"("Name"="Auto Selector") -> ("String"=w44:string)  [unwired: 9 in, 1 out]
  n21 = String Subset(string=w41, offset (0)=0, length (rest)=1 ("length (rest)")) -> (substring=w37:string)
  n22 = call-poly <vilib>:"NT Write Value.vi"("Numeric Array"=w43, "Name"="Joystick 0/Axes") -> ()  [unwired: 9 in, 1 out]
  n23 = Index Array(array=w43, index=2) -> ()  [unwired: 1 out]
  n24 = case shown="\"CENTER\"" w44 {
    tunnel: "1" -> [w61 w478 _ _ _ _]
    tunnel: w37 -> [w60 w477 _ _ _ _]
    tunnel: w25 -> [w59 w476 _ _ _ _]
    tunnel: w24 -> [w58 w475 _ _ _ _]
    tunnel: w27 -> [w57 w474 _ _ _ _]
    tunnel: w26 -> [w56 w473 _ _ _ _]
    tunnel: w28 -> [w55 w472 _ _ _ _]
    tunnel: w29 -> [w54 w471 _ _ _ _]
    tunnel: w31 -> [w53 w470 _ _ _ _]
    tunnel: w3 -> [w52 w469 _ _ _ _]
    frame "CENTER" {
      n25 = while {
        shift-right: [w74] -> _
        shift-left: w60 -> [w73]
        shift-right: [w72] -> _
        shift-left: w61 -> [w71]
        tunnel: w59 -> [w69]
        tunnel: w58 -> [w68]
        tunnel: w57 -> [w67]
        tunnel: w56 -> [w66]
        tunnel: w55 -> [w65]
        tunnel: w54 -> [w64]
        tunnel: w53 -> [w63]
        tunnel: w52 -> [w62]
        stop <- w70 stop-if-true
        n26 = case shown="\"R\", Default" w73 {
          selector: w73 -> [w84 w149]
          tunnel: [w83 w150] -> w74
          tunnel: [w87 w146] -> w72
          tunnel: w71 -> [w85 w148]
          tunnel: [w86 w147] -> w70
          tunnel: w69 -> [w78 w145]
          tunnel: w68 -> [w77 w144]
          tunnel: w67 -> [w76 w143]
          tunnel: w66 -> [w82 w142]
          tunnel: w65 -> [w79 w141]
          tunnel: w64 -> [w80 w140]
          tunnel: w63 -> [w81 w139]
          tunnel: w62 -> [w75 w138]
          frame "L" {
            (unwired) TRUE
            n27 = case shown="\"1 \", Default" w85 {
              tunnel: ["4" ("t") "\"4\"" ("t") w105 "3" ("t")] -> w87
              tunnel: [FALSE TRUE FALSE FALSE] -> w86
              tunnel: w84 -> [w89 w91 w133 w136]
              tunnel: [w89 w91 w133 w136] -> w83
              tunnel: w82 -> [_ _ w128 _]
              tunnel: w81 -> [_ _ w127 _]
              tunnel: w80 -> [_ _ w126 _]
              tunnel: w79 -> [_ _ w125 _]
              tunnel: w78 -> [_ _ w124 _]
              tunnel: w77 -> [_ _ w123 _]
              tunnel: w76 -> [_ _ w122 _]
              tunnel: w75 -> [_ _ w94 _]
              frame "3" {
              }
              frame "4" {
              }
              frame "1 ", Default {
                w98 = T9 0 items=["PercentOutput"=0, "Position"=1, "Velocity"=2, "Current"=3, "Follower"=5, "MotionProfile"=6, "MotionMagic"=7, "MotionMagicArc"=8, "MotionProfileArc"=10, "Disabled"=15] ("Control Mode")
                w99 = T9 0 items=["PercentOutput"=0, "Position"=1, "Velocity"=2, "Current"=3, "Follower"=5, "MotionProfile"=6, "MotionMagic"=7, "MotionMagicArc"=8, "MotionProfileArc"=10, "Disabled"=15] ("Control Mode")
                w129 = T9 7 items=["PercentOutput"=0, "Position"=1, "Velocity"=2, "Current"=3, "Follower"=5, "MotionProfile"=6, "MotionMagic"=7, "MotionMagicArc"=8, "MotionProfileArc"=10, "Disabled"=15] ("Control Mode")
                w130 = T9 7 items=["PercentOutput"=0, "Position"=1, "Velocity"=2, "Current"=3, "Follower"=5, "MotionProfile"=6, "MotionMagic"=7, "MotionMagicArc"=8, "MotionProfileArc"=10, "Disabled"=15] ("Control Mode")
                w131 = T9 0 items=["PercentOutput"=0, "Position"=1, "Velocity"=2, "Current"=3, "Follower"=5, "MotionProfile"=6, "MotionMagic"=7, "MotionMagicArc"=8, "MotionProfileArc"=10, "Disabled"=15] ("Control Mode")
                w132 = T9 0 items=["PercentOutput"=0, "Position"=1, "Velocity"=2, "Current"=3, "Follower"=5, "MotionProfile"=6, "MotionMagic"=7, "MotionMagicArc"=8, "MotionProfileArc"=10, "Disabled"=15] ("Control Mode")
                n28 = call <vilib>:"CTRE_Phoenix_MotorControl_Set.vi"("error in (no error)"=w127, "Output"="Lt Target 1", "Control Mode"=w129, "PhoenixMotorControlDevRef"=w94) -> ("error out"=w115:errorcluster, "PhoenixMotorControlDevRef"=w116:T2)  [unwired: 6 in]
                n29 = call <vilib>:"CTRE_Phoenix_MotorControl_Set.vi"("error in (no error)"=w125, "Output"="Lt Target 1", "Control Mode"=w130, "PhoenixMotorControlDevRef"=w126) -> ("error out"=w117:errorcluster, "PhoenixMotorControlDevRef"=w118:T2)  [unwired: 6 in]
                n30 = call <vilib>:"CTRE_Phoenix_MotorControl_Set.vi"("error in (no error)"=w128, "Output"=0.0, "Control Mode"=w131, "PhoenixMotorControlDevRef"=w122) -> ()  [unwired: 6 in, 2 out]
                n31 = call <vilib>:"CTRE_Phoenix_MotorControl_Set.vi"("error in (no error)"=w123, "Output"=0.0, "Control Mode"=w132, "PhoenixMotorControlDevRef"=w124) -> ()  [unwired: 6 in, 2 out]
                n32 = call-poly <vilib>:"CTRE_Phoenix_MotorController_Get_Enhanced.vi"("PhoenixMotorControlDevRef"=w116, "error in"=w115) -> ("PhoenixMotorControlDevRef"=w101:T2, "Closed-loop Error"=w114:i32, "error out"=w100:errorcluster)  [unwired: 8 in, 3 out]
                "Closed-loop Error RF" <- w114
                n33 = call-poly <vilib>:"CTRE_Phoenix_MotorController_Get_Enhanced.vi"("PhoenixMotorControlDevRef"=w118, "error in"=w117) -> ("PhoenixMotorControlDevRef"=w97:T2, "Closed-loop Error"=w113:i32, "error out"=w96:errorcluster)  [unwired: 8 in, 3 out]
                "Closed-loop Error LR" <- w113
                n34 = call <vilib>:"CTRE_Phoenix_MotorControl_Set.vi"("error in (no error)"=w100, "Output"=0.0, "Control Mode"=w99, "PhoenixMotorControlDevRef"=w101) -> ()  [unwired: 6 in, 2 out]
                n35 = call <vilib>:"CTRE_Phoenix_MotorControl_Set.vi"("error in (no error)"=w96, "Output"=0.0, "Control Mode"=w98, "PhoenixMotorControlDevRef"=w97) -> ()  [unwired: 6 in, 2 out]
                n36 = Absolute Value(x=w114) -> (abs(x)=w110:i32)
                n37 = Absolute Value(x=w113) -> (abs(x)=w109:i32)
                n38 = Add(x=w110, y=w109) -> (x+y=w112:i32)
                n39 = Divide(x=w112, y=2) -> (x/y=w108:dbl)
                n40 = Greater?(x=w108, y=200.0) -> (0:w106:bool)
                n41 = Select(t="1", s=w106, f="2") -> (s? t:f=w105:string)
              }
              frame "2" {
              }
            }
          }
          frame "R", Default {
            n42 = case shown="\"1 \", Default" w148 {
              tunnel: w149 -> [w191 w207 w242 w258 w292 w308 w348 w364 w398 w414 w448 w466]
              tunnel: [w191 w207 w242 w258 w292 w308 w348 w364 w398 w414 w448 w466] -> w150
              tunnel: [w186 "3" ("f") w240 "5" ("f") w290 "7" ("f") w343 "9" ("f") w396 "11" ("f") w446 "8" ("t")] -> w146
              tunnel: [FALSE FALSE FALSE FALSE FALSE FALSE FALSE FALSE FALSE FALSE FALSE TRUE] -> w147
              tunnel: w145 -> [w185 w201 w216 w252 w266 w302 w342 w358 w372 w408 w422 w465]
              tunnel: w144 -> [w184 w200 w215 w251 w265 w301 w341 w357 w371 w407 w421 w464]
              tunnel: w143 -> [w183 w198 w213 w249 w263 w299 w340 w355 w369 w405 w419 w463]
              tunnel: w142 -> [w182 w199 w214 w250 w264 w300 w339 w356 w370 w406 w420 w462]
              tunnel: w141 -> [w189 w197 w212 w248 w262 w298 w346 w354 w368 w404 w418 w453]
              tunnel: w140 -> [w188 w196 w211 w247 w261 w297 w345 w353 w367 w403 w417 w452]
              tunnel: w139 -> [w187 w194 w209 w245 w259 w295 w344 w351 w365 w401 w415 w451]
              tunnel: w138 -> [w181 w195 w210 w246 w260 w296 w338 w352 w366 w402 w416 w450]
              frame "1 ", Default {
                w161 = 36500.0 ("RT Target")
                w162 = 0.0 ("Lt Target 2")
                w163 = T9 0 items=["PercentOutput"=0, "Position"=1, "Velocity"=2, "Current"=3, "Follower"=5, "MotionProfile"=6, "MotionMagic"=7, "MotionMagicArc"=8, "MotionProfileArc"=10, "Disabled"=15] ("Control Mode")
                w164 = T9 0 items=["PercentOutput"=0, "Position"=1, "Velocity"=2, "Current"=3, "Follower"=5, "MotionProfile"=6, "MotionMagic"=7, "MotionMagicArc"=8, "MotionProfileArc"=10, "Disabled"=15] ("Control Mode")
                w165 = T9 7 items=["PercentOutput"=0, "Position"=1, "Velocity"=2, "Current"=3, "Follower"=5, "MotionProfile"=6, "MotionMagic"=7, "MotionMagicArc"=8, "MotionProfileArc"=10, "Disabled"=15] ("Control Mode")
                w166 = T9 7 items=["PercentOutput"=0, "Position"=1, "Velocity"=2, "Current"=3, "Follower"=5, "MotionProfile"=6, "MotionMagic"=7, "MotionMagicArc"=8, "MotionProfileArc"=10, "Disabled"=15] ("Control Mode")
                n43 = Wait (ms)(milliseconds to wait=u32 4500) -> ()  [unwired: 1 out]
                n44 = call <vilib>:"CTRE_Phoenix_MotorControl_ConfigAllowableClosedLoopError.vi"("error in (no error)"=w182, "slotIdx"=u32 0, "allowableClosedLoopError"=200, "PhoenixMotorControlDevRef"=w183) -> ("error out"=w155:errorcluster, "PhoenixMotorControlDevRef"=w156:T2)  [unwired: 6 in]
                n45 = call <vilib>:"CTRE_Phoenix_MotorControl_ConfigAllowableClosedLoopError.vi"("error in (no error)"=w184, "slotIdx"=u32 0, "allowableClosedLoopError"=200, "PhoenixMotorControlDevRef"=w185) -> ("error out"=w159:errorcluster, "PhoenixMotorControlDevRef"=w160:T2)  [unwired: 6 in]
                n46 = call <vilib>:"CTRE_Phoenix_MotorControl_Set.vi"("error in (no error)"=w155, "Output"=w161, "Control Mode"=w165, "PhoenixMotorControlDevRef"=w156) -> ("error out"=w169:errorcluster, "PhoenixMotorControlDevRef"=w170:T2)  [unwired: 6 in]
                n47 = call <vilib>:"CTRE_Phoenix_MotorControl_Set.vi"("error in (no error)"=w187, "Output"=w162, "Control Mode"=w163, "PhoenixMotorControlDevRef"=w181) -> ()  [unwired: 6 in, 2 out]
                n48 = call <vilib>:"CTRE_Phoenix_MotorControl_Set.vi"("error in (no error)"=w189, "Output"=w162, "Control Mode"=w164, "PhoenixMotorControlDevRef"=w188) -> ()  [unwired: 6 in, 2 out]
                n49 = call <vilib>:"CTRE_Phoenix_MotorControl_Set.vi"("error in (no error)"=w159, "Output"=w161, "Control Mode"=w166, "PhoenixMotorControlDevRef"=w160) -> ("error out"=w167:errorcluster, "PhoenixMotorControlDevRef"=w168:T2)  [unwired: 6 in]
                n50 = call-poly <vilib>:"CTRE_Phoenix_MotorController_Get_Enhanced.vi"("PhoenixMotorControlDevRef"=w168, "error in"=w167) -> ("Closed-loop Error"=w179:i32)  [unwired: 8 in, 5 out]
                n51 = call-poly <vilib>:"CTRE_Phoenix_MotorController_Get_Enhanced.vi"("PhoenixMotorControlDevRef"=w170, "error in"=w169) -> ("Closed-loop Error"=w180:i32)  [unwired: 8 in, 5 out]
                n52 = Absolute Value(x=w180) -> (abs(x)=w176:i32)
                n53 = Absolute Value(x=w179) -> (abs(x)=w175:i32)
                n54 = Add(x=w176, y=w175) -> (x+y=w178:i32)
                n55 = Divide(x=w178, y=2) -> (x/y=w174:dbl)
                n56 = Greater?(x=w174, y=200.0) -> (0:w152:bool)
                n57 = Select(t="1", s=w152, f="2") -> (s? t:f=w186:string)
              }
              frame "2" {
                w193 = u32 10 ("timeoutMs")
                n58 = call <vilib>:"CTRE_Phoenix_MotorControl_SetSelectedSensorPosition.vi"("timeoutMs"=w193, "error in (no error)"=w194, "New Sensor Position"=0, "PhoenixMotorControlDevRef"=w195) -> ()  [unwired: 6 in, 2 out]
                n59 = call <vilib>:"CTRE_Phoenix_MotorControl_SetSelectedSensorPosition.vi"("timeoutMs"=w193, "error in (no error)"=w200, "New Sensor Position"=0, "PhoenixMotorControlDevRef"=w201) -> ()  [unwired: 6 in, 2 out]
                n60 = call <vilib>:"CTRE_Phoenix_MotorControl_SetSelectedSensorPosition.vi"("timeoutMs"=w193, "error in (no error)"=w197, "New Sensor Position"=0, "PhoenixMotorControlDevRef"=w196) -> ()  [unwired: 6 in, 2 out]
                n61 = call <vilib>:"CTRE_Phoenix_MotorControl_SetSelectedSensorPosition.vi"("timeoutMs"=w193, "error in (no error)"=w199, "New Sensor Position"=0, "PhoenixMotorControlDevRef"=w198) -> ()  [unwired: 6 in, 2 out]
              }
              frame "3" {
                w221 = T9 7 items=["PercentOutput"=0, "Position"=1, "Velocity"=2, "Current"=3, "Follower"=5, "MotionProfile"=6, "MotionMagic"=7, "MotionMagicArc"=8, "MotionProfileArc"=10, "Disabled"=15] ("Control Mode")
                w222 = T9 7 items=["PercentOutput"=0, "Position"=1, "Velocity"=2, "Current"=3, "Follower"=5, "MotionProfile"=6, "MotionMagic"=7, "MotionMagicArc"=8, "MotionProfileArc"=10, "Disabled"=15] ("Control Mode")
                w238 = T9 7 items=["PercentOutput"=0, "Position"=1, "Velocity"=2, "Current"=3, "Follower"=5, "MotionProfile"=6, "MotionMagic"=7, "MotionMagicArc"=8, "MotionProfileArc"=10, "Disabled"=15] ("Control Mode")
                w239 = T9 7 items=["PercentOutput"=0, "Position"=1, "Velocity"=2, "Current"=3, "Follower"=5, "MotionProfile"=6, "MotionMagic"=7, "MotionMagicArc"=8, "MotionProfileArc"=10, "Disabled"=15] ("Control Mode")
                n62 = Wait (ms)(milliseconds to wait=u32 1500) -> ()  [unwired: 1 out]
                n63 = call <vilib>:"CTRE_Phoenix_MotorControl_Set.vi"("error in (no error)"=w214, "Output"=3500.0, "Control Mode"=w238, "PhoenixMotorControlDevRef"=w213) -> ("error out"=w226:errorcluster, "PhoenixMotorControlDevRef"=w227:T2)  [unwired: 6 in]
                n64 = call <vilib>:"CTRE_Phoenix_MotorControl_Set.vi"("error in (no error)"=w215, "Output"=3500.0, "Control Mode"=w239, "PhoenixMotorControlDevRef"=w216) -> ("error out"=w224:errorcluster, "PhoenixMotorControlDevRef"=w225:T2)  [unwired: 6 in]
                n65 = call <vilib>:"CTRE_Phoenix_MotorControl_Set.vi"("error in (no error)"=w209, "Output"=-3500.0, "Control Mode"=w221, "PhoenixMotorControlDevRef"=w210) -> ()  [unwired: 6 in, 2 out]
                n66 = call <vilib>:"CTRE_Phoenix_MotorControl_Set.vi"("error in (no error)"=w212, "Output"=-3500.0, "Control Mode"=w222, "PhoenixMotorControlDevRef"=w211) -> ()  [unwired: 6 in, 2 out]
                n67 = call-poly <vilib>:"CTRE_Phoenix_MotorController_Get_Enhanced.vi"("PhoenixMotorControlDevRef"=w227, "error in"=w226) -> ("Closed-loop Error"=w237:i32)  [unwired: 8 in, 5 out]
                n68 = call-poly <vilib>:"CTRE_Phoenix_MotorController_Get_Enhanced.vi"("PhoenixMotorControlDevRef"=w225, "error in"=w224) -> ("Closed-loop Error"=w236:i32)  [unwired: 8 in, 5 out]
                n69 = Absolute Value(x=w237) -> (abs(x)=w233:i32)
                n70 = Absolute Value(x=w236) -> (abs(x)=w232:i32)
                n71 = Add(x=w233, y=w232) -> (x+y=w235:i32)
                n72 = Divide(x=w235, y=2) -> (x/y=w231:dbl)
                n73 = Greater?(x=w231, y=200.0) -> (0:w223:bool)
                n74 = Select(t="3", s=w223, f="12") -> (s? t:f=w240:string)
              }
              frame "4" {
                w244 = u32 10 ("timeoutMs")
                n75 = call <vilib>:"CTRE_Phoenix_MotorControl_SetSelectedSensorPosition.vi"("timeoutMs"=w244, "error in (no error)"=w245, "New Sensor Position"=0, "PhoenixMotorControlDevRef"=w246) -> ()  [unwired: 6 in, 2 out]
                n76 = call <vilib>:"CTRE_Phoenix_MotorControl_SetSelectedSensorPosition.vi"("timeoutMs"=w244, "error in (no error)"=w251, "New Sensor Position"=0, "PhoenixMotorControlDevRef"=w252) -> ()  [unwired: 6 in, 2 out]
                n77 = call <vilib>:"CTRE_Phoenix_MotorControl_SetSelectedSensorPosition.vi"("timeoutMs"=w244, "error in (no error)"=w248, "New Sensor Position"=0, "PhoenixMotorControlDevRef"=w247) -> ()  [unwired: 6 in, 2 out]
                n78 = call <vilib>:"CTRE_Phoenix_MotorControl_SetSelectedSensorPosition.vi"("timeoutMs"=w244, "error in (no error)"=w250, "New Sensor Position"=0, "PhoenixMotorControlDevRef"=w249) -> ()  [unwired: 6 in, 2 out]
              }
              frame "5" {
                w271 = T9 7 items=["PercentOutput"=0, "Position"=1, "Velocity"=2, "Current"=3, "Follower"=5, "MotionProfile"=6, "MotionMagic"=7, "MotionMagicArc"=8, "MotionProfileArc"=10, "Disabled"=15] ("Control Mode")
                w272 = T9 7 items=["PercentOutput"=0, "Position"=1, "Velocity"=2, "Current"=3, "Follower"=5, "MotionProfile"=6, "MotionMagic"=7, "MotionMagicArc"=8, "MotionProfileArc"=10, "Disabled"=15] ("Control Mode")
                w288 = T9 7 items=["PercentOutput"=0, "Position"=1, "Velocity"=2, "Current"=3, "Follower"=5, "MotionProfile"=6, "MotionMagic"=7, "MotionMagicArc"=8, "MotionProfileArc"=10, "Disabled"=15] ("Control Mode")
                w289 = T9 7 items=["PercentOutput"=0, "Position"=1, "Velocity"=2, "Current"=3, "Follower"=5, "MotionProfile"=6, "MotionMagic"=7, "MotionMagicArc"=8, "MotionProfileArc"=10, "Disabled"=15] ("Control Mode")
                n79 = call <vilib>:"CTRE_Phoenix_MotorControl_Set.vi"("error in (no error)"=w264, "Output"=-3500.0, "Control Mode"=w288, "PhoenixMotorControlDevRef"=w263) -> ("error out"=w276:errorcluster, "PhoenixMotorControlDevRef"=w277:T2)  [unwired: 6 in]
                n80 = call <vilib>:"CTRE_Phoenix_MotorControl_Set.vi"("error in (no error)"=w265, "Output"=-3500.0, "Control Mode"=w289, "PhoenixMotorControlDevRef"=w266) -> ("error out"=w274:errorcluster, "PhoenixMotorControlDevRef"=w275:T2)  [unwired: 6 in]
                n81 = call <vilib>:"CTRE_Phoenix_MotorControl_Set.vi"("error in (no error)"=w259, "Output"=3500.0, "Control Mode"=w271, "PhoenixMotorControlDevRef"=w260) -> ()  [unwired: 6 in, 2 out]
                n82 = call <vilib>:"CTRE_Phoenix_MotorControl_Set.vi"("error in (no error)"=w262, "Output"=3500.0, "Control Mode"=w272, "PhoenixMotorControlDevRef"=w261) -> ()  [unwired: 6 in, 2 out]
                n83 = call-poly <vilib>:"CTRE_Phoenix_MotorController_Get_Enhanced.vi"("PhoenixMotorControlDevRef"=w277, "error in"=w276) -> ("Closed-loop Error"=w287:i32)  [unwired: 8 in, 5 out]
                n84 = call-poly <vilib>:"CTRE_Phoenix_MotorController_Get_Enhanced.vi"("PhoenixMotorControlDevRef"=w275, "error in"=w274) -> ("Closed-loop Error"=w286:i32)  [unwired: 8 in, 5 out]
                n85 = Absolute Value(x=w287) -> (abs(x)=w283:i32)
                n86 = Absolute Value(x=w286) -> (abs(x)=w282:i32)
                n87 = Add(x=w283, y=w282) -> (x+y=w285:i32)
                n88 = Divide(x=w285, y=2) -> (x/y=w281:dbl)
                n89 = Greater?(x=w281, y=200.0) -> (0:w273:bool)
                n90 = Select(t="5", s=w273, f="6") -> (s? t:f=w290:string)
              }
              frame "6" {
                w294 = u32 10 ("timeoutMs")
                n91 = call <vilib>:"CTRE_Phoenix_MotorControl_SetSelectedSensorPosition.vi"("timeoutMs"=w294, "error in (no error)"=w295, "New Sensor Position"=0, "PhoenixMotorControlDevRef"=w296) -> ()  [unwired: 6 in, 2 out]
                n92 = call <vilib>:"CTRE_Phoenix_MotorControl_SetSelectedSensorPosition.vi"("timeoutMs"=w294, "error in (no error)"=w301, "New Sensor Position"=0, "PhoenixMotorControlDevRef"=w302) -> ()  [unwired: 6 in, 2 out]
                n93 = call <vilib>:"CTRE_Phoenix_MotorControl_SetSelectedSensorPosition.vi"("timeoutMs"=w294, "error in (no error)"=w298, "New Sensor Position"=0, "PhoenixMotorControlDevRef"=w297) -> ()  [unwired: 6 in, 2 out]
                n94 = call <vilib>:"CTRE_Phoenix_MotorControl_SetSelectedSensorPosition.vi"("timeoutMs"=w294, "error in (no error)"=w300, "New Sensor Position"=0, "PhoenixMotorControlDevRef"=w299) -> ()  [unwired: 6 in, 2 out]
              }
              frame "7" {
                w318 = -36500.0 ("RT Target")
                w319 = 0.0 ("Lt Target 2")
                w320 = T9 0 items=["PercentOutput"=0, "Position"=1, "Velocity"=2, "Current"=3, "Follower"=5, "MotionProfile"=6, "MotionMagic"=7, "MotionMagicArc"=8, "MotionProfileArc"=10, "Disabled"=15] ("Control Mode")
                w321 = T9 0 items=["PercentOutput"=0, "Position"=1, "Velocity"=2, "Current"=3, "Follower"=5, "MotionProfile"=6, "MotionMagic"=7, "MotionMagicArc"=8, "MotionProfileArc"=10, "Disabled"=15] ("Control Mode")
                w322 = T9 7 items=["PercentOutput"=0, "Position"=1, "Velocity"=2, "Current"=3, "Follower"=5, "MotionProfile"=6, "MotionMagic"=7, "MotionMagicArc"=8, "MotionProfileArc"=10, "Disabled"=15] ("Control Mode")
                w323 = T9 7 items=["PercentOutput"=0, "Position"=1, "Velocity"=2, "Current"=3, "Follower"=5, "MotionProfile"=6, "MotionMagic"=7, "MotionMagicArc"=8, "MotionProfileArc"=10, "Disabled"=15] ("Control Mode")
                n95 = call <vilib>:"CTRE_Phoenix_MotorControl_ConfigAllowableClosedLoopError.vi"("error in (no error)"=w339, "slotIdx"=u32 0, "allowableClosedLoopError"=200, "PhoenixMotorControlDevRef"=w340) -> ("error out"=w312:errorcluster, "PhoenixMotorControlDevRef"=w313:T2)  [unwired: 6 in]
                n96 = call <vilib>:"CTRE_Phoenix_MotorControl_ConfigAllowableClosedLoopError.vi"("error in (no error)"=w341, "slotIdx"=u32 0, "allowableClosedLoopError"=200, "PhoenixMotorControlDevRef"=w342) -> ("error out"=w316:errorcluster, "PhoenixMotorControlDevRef"=w317:T2)  [unwired: 6 in]
                n97 = call <vilib>:"CTRE_Phoenix_MotorControl_Set.vi"("error in (no error)"=w312, "Output"=w318, "Control Mode"=w322, "PhoenixMotorControlDevRef"=w313) -> ("error out"=w326:errorcluster, "PhoenixMotorControlDevRef"=w327:T2)  [unwired: 6 in]
                n98 = call <vilib>:"CTRE_Phoenix_MotorControl_Set.vi"("error in (no error)"=w344, "Output"=w319, "Control Mode"=w320, "PhoenixMotorControlDevRef"=w338) -> ()  [unwired: 6 in, 2 out]
                n99 = call <vilib>:"CTRE_Phoenix_MotorControl_Set.vi"("error in (no error)"=w346, "Output"=w319, "Control Mode"=w321, "PhoenixMotorControlDevRef"=w345) -> ()  [unwired: 6 in, 2 out]
                n100 = call <vilib>:"CTRE_Phoenix_MotorControl_Set.vi"("error in (no error)"=w316, "Output"=w318, "Control Mode"=w323, "PhoenixMotorControlDevRef"=w317) -> ("error out"=w324:errorcluster, "PhoenixMotorControlDevRef"=w325:T2)  [unwired: 6 in]
                n101 = call-poly <vilib>:"CTRE_Phoenix_MotorController_Get_Enhanced.vi"("PhoenixMotorControlDevRef"=w325, "error in"=w324) -> ("Closed-loop Error"=w336:i32)  [unwired: 8 in, 5 out]
                n102 = call-poly <vilib>:"CTRE_Phoenix_MotorController_Get_Enhanced.vi"("PhoenixMotorControlDevRef"=w327, "error in"=w326) -> ("Closed-loop Error"=w337:i32)  [unwired: 8 in, 5 out]
                n103 = Absolute Value(x=w337) -> (abs(x)=w333:i32)
                n104 = Absolute Value(x=w336) -> (abs(x)=w332:i32)
                n105 = Add(x=w333, y=w332) -> (x+y=w335:i32)
                n106 = Divide(x=w335, y=2) -> (x/y=w331:dbl)
                n107 = Greater?(x=w331, y=200.0) -> (0:w309:bool)
                n108 = Select(t="7", s=w309, f="8") -> (s? t:f=w343:string)
              }
              frame "8" {
                w350 = u32 10 ("timeoutMs")
                n109 = call <vilib>:"CTRE_Phoenix_MotorControl_SetSelectedSensorPosition.vi"("timeoutMs"=w350, "error in (no error)"=w351, "New Sensor Position"=0, "PhoenixMotorControlDevRef"=w352) -> ()  [unwired: 6 in, 2 out]
                n110 = call <vilib>:"CTRE_Phoenix_MotorControl_SetSelectedSensorPosition.vi"("timeoutMs"=w350, "error in (no error)"=w357, "New Sensor Position"=0, "PhoenixMotorControlDevRef"=w358) -> ()  [unwired: 6 in, 2 out]
                n111 = call <vilib>:"CTRE_Phoenix_MotorControl_SetSelectedSensorPosition.vi"("timeoutMs"=w350, "error in (no error)"=w354, "New Sensor Position"=0, "PhoenixMotorControlDevRef"=w353) -> ()  [unwired: 6 in, 2 out]
                n112 = call <vilib>:"CTRE_Phoenix_MotorControl_SetSelectedSensorPosition.vi"("timeoutMs"=w350, "error in (no error)"=w356, "New Sensor Position"=0, "PhoenixMotorControlDevRef"=w355) -> ()  [unwired: 6 in, 2 out]
              }
              frame "9" {
                w377 = T9 7 items=["PercentOutput"=0, "Position"=1, "Velocity"=2, "Current"=3, "Follower"=5, "MotionProfile"=6, "MotionMagic"=7, "MotionMagicArc"=8, "MotionProfileArc"=10, "Disabled"=15] ("Control Mode")
                w378 = T9 7 items=["PercentOutput"=0, "Position"=1, "Velocity"=2, "Current"=3, "Follower"=5, "MotionProfile"=6, "MotionMagic"=7, "MotionMagicArc"=8, "MotionProfileArc"=10, "Disabled"=15] ("Control Mode")
                w394 = T9 7 items=["PercentOutput"=0, "Position"=1, "Velocity"=2, "Current"=3, "Follower"=5, "MotionProfile"=6, "MotionMagic"=7, "MotionMagicArc"=8, "MotionProfileArc"=10, "Disabled"=15] ("Control Mode")
                w395 = T9 7 items=["PercentOutput"=0, "Position"=1, "Velocity"=2, "Current"=3, "Follower"=5, "MotionProfile"=6, "MotionMagic"=7, "MotionMagicArc"=8, "MotionProfileArc"=10, "Disabled"=15] ("Control Mode")
                n113 = call <vilib>:"CTRE_Phoenix_MotorControl_Set.vi"("error in (no error)"=w370, "Output"=-1500.0, "Control Mode"=w394, "PhoenixMotorControlDevRef"=w369) -> ("error out"=w382:errorcluster, "PhoenixMotorControlDevRef"=w383:T2)  [unwired: 6 in]
                n114 = call <vilib>:"CTRE_Phoenix_MotorControl_Set.vi"("error in (no error)"=w371, "Output"=-1500.0, "Control Mode"=w395, "PhoenixMotorControlDevRef"=w372) -> ("error out"=w380:errorcluster, "PhoenixMotorControlDevRef"=w381:T2)  [unwired: 6 in]
                n115 = call <vilib>:"CTRE_Phoenix_MotorControl_Set.vi"("error in (no error)"=w365, "Output"=1500.0, "Control Mode"=w377, "PhoenixMotorControlDevRef"=w366) -> ()  [unwired: 6 in, 2 out]
                n116 = call <vilib>:"CTRE_Phoenix_MotorControl_Set.vi"("error in (no error)"=w368, "Output"=1500.0, "Control Mode"=w378, "PhoenixMotorControlDevRef"=w367) -> ()  [unwired: 6 in, 2 out]
                n117 = call-poly <vilib>:"CTRE_Phoenix_MotorController_Get_Enhanced.vi"("PhoenixMotorControlDevRef"=w383, "error in"=w382) -> ("Closed-loop Error"=w393:i32)  [unwired: 8 in, 5 out]
                n118 = call-poly <vilib>:"CTRE_Phoenix_MotorController_Get_Enhanced.vi"("PhoenixMotorControlDevRef"=w381, "error in"=w380) -> ("Closed-loop Error"=w392:i32)  [unwired: 8 in, 5 out]
                n119 = Absolute Value(x=w393) -> (abs(x)=w389:i32)
                n120 = Absolute Value(x=w392) -> (abs(x)=w388:i32)
                n121 = Add(x=w389, y=w388) -> (x+y=w391:i32)
                n122 = Divide(x=w391, y=2) -> (x/y=w387:dbl)
                n123 = Greater?(x=w387, y=200.0) -> (0:w379:bool)
                n124 = Select(t="9", s=w379, f="10") -> (s? t:f=w396:string)
              }
              frame "10" {
                w400 = u32 10 ("timeoutMs")
                n125 = call <vilib>:"CTRE_Phoenix_MotorControl_SetSelectedSensorPosition.vi"("timeoutMs"=w400, "error in (no error)"=w401, "New Sensor Position"=0, "PhoenixMotorControlDevRef"=w402) -> ()  [unwired: 6 in, 2 out]
                n126 = call <vilib>:"CTRE_Phoenix_MotorControl_SetSelectedSensorPosition.vi"("timeoutMs"=w400, "error in (no error)"=w407, "New Sensor Position"=0, "PhoenixMotorControlDevRef"=w408) -> ()  [unwired: 6 in, 2 out]
                n127 = call <vilib>:"CTRE_Phoenix_MotorControl_SetSelectedSensorPosition.vi"("timeoutMs"=w400, "error in (no error)"=w404, "New Sensor Position"=0, "PhoenixMotorControlDevRef"=w403) -> ()  [unwired: 6 in, 2 out]
                n128 = call <vilib>:"CTRE_Phoenix_MotorControl_SetSelectedSensorPosition.vi"("timeoutMs"=w400, "error in (no error)"=w406, "New Sensor Position"=0, "PhoenixMotorControlDevRef"=w405) -> ()  [unwired: 6 in, 2 out]
              }
              frame "11" {
                w427 = T9 7 items=["PercentOutput"=0, "Position"=1, "Velocity"=2, "Current"=3, "Follower"=5, "MotionProfile"=6, "MotionMagic"=7, "MotionMagicArc"=8, "MotionProfileArc"=10, "Disabled"=15] ("Control Mode")
                w428 = T9 7 items=["PercentOutput"=0, "Position"=1, "Velocity"=2, "Current"=3, "Follower"=5, "MotionProfile"=6, "MotionMagic"=7, "MotionMagicArc"=8, "MotionProfileArc"=10, "Disabled"=15] ("Control Mode")
                w444 = T9 7 items=["PercentOutput"=0, "Position"=1, "Velocity"=2, "Current"=3, "Follower"=5, "MotionProfile"=6, "MotionMagic"=7, "MotionMagicArc"=8, "MotionProfileArc"=10, "Disabled"=15] ("Control Mode")
                w445 = T9 7 items=["PercentOutput"=0, "Position"=1, "Velocity"=2, "Current"=3, "Follower"=5, "MotionProfile"=6, "MotionMagic"=7, "MotionMagicArc"=8, "MotionProfileArc"=10, "Disabled"=15] ("Control Mode")
                n129 = call <vilib>:"CTRE_Phoenix_MotorControl_Set.vi"("error in (no error)"=w420, "Output"=1500.0, "Control Mode"=w444, "PhoenixMotorControlDevRef"=w419) -> ("error out"=w432:errorcluster, "PhoenixMotorControlDevRef"=w433:T2)  [unwired: 6 in]
                n130 = call <vilib>:"CTRE_Phoenix_MotorControl_Set.vi"("error in (no error)"=w421, "Output"=1500.0, "Control Mode"=w445, "PhoenixMotorControlDevRef"=w422) -> ("error out"=w430:errorcluster, "PhoenixMotorControlDevRef"=w431:T2)  [unwired: 6 in]
                n131 = call <vilib>:"CTRE_Phoenix_MotorControl_Set.vi"("error in (no error)"=w415, "Output"=1500.0, "Control Mode"=w427, "PhoenixMotorControlDevRef"=w416) -> ()  [unwired: 6 in, 2 out]
                n132 = call <vilib>:"CTRE_Phoenix_MotorControl_Set.vi"("error in (no error)"=w418, "Output"=1500.0, "Control Mode"=w428, "PhoenixMotorControlDevRef"=w417) -> ()  [unwired: 6 in, 2 out]
                n133 = call-poly <vilib>:"CTRE_Phoenix_MotorController_Get_Enhanced.vi"("PhoenixMotorControlDevRef"=w433, "error in"=w432) -> ("Closed-loop Error"=w443:i32)  [unwired: 8 in, 5 out]
                n134 = call-poly <vilib>:"CTRE_Phoenix_MotorController_Get_Enhanced.vi"("PhoenixMotorControlDevRef"=w431, "error in"=w430) -> ("Closed-loop Error"=w442:i32)  [unwired: 8 in, 5 out]
                n135 = Absolute Value(x=w443) -> (abs(x)=w439:i32)
                n136 = Absolute Value(x=w442) -> (abs(x)=w438:i32)
                n137 = Add(x=w439, y=w438) -> (x+y=w441:i32)
                n138 = Divide(x=w441, y=2) -> (x/y=w437:dbl)
                n139 = Greater?(x=w437, y=200.0) -> (0:w429:bool)
                n140 = Select(t="11", s=w429, f="12") -> (s? t:f=w446:string)
              }
              frame "12" {
                w455 = T9 0 items=["PercentOutput"=0, "Position"=1, "Velocity"=2, "Current"=3, "Follower"=5, "MotionProfile"=6, "MotionMagic"=7, "MotionMagicArc"=8, "MotionProfileArc"=10, "Disabled"=15] ("Control Mode")
                w457 = T9 0 items=["PercentOutput"=0, "Position"=1, "Velocity"=2, "Current"=3, "Follower"=5, "MotionProfile"=6, "MotionMagic"=7, "MotionMagicArc"=8, "MotionProfileArc"=10, "Disabled"=15] ("Control Mode")
                w459 = T9 0 items=["PercentOutput"=0, "Position"=1, "Velocity"=2, "Current"=3, "Follower"=5, "MotionProfile"=6, "MotionMagic"=7, "MotionMagicArc"=8, "MotionProfileArc"=10, "Disabled"=15] ("Control Mode")
                w461 = T9 0 items=["PercentOutput"=0, "Position"=1, "Velocity"=2, "Current"=3, "Follower"=5, "MotionProfile"=6, "MotionMagic"=7, "MotionMagicArc"=8, "MotionProfileArc"=10, "Disabled"=15] ("Control Mode")
                n141 = call <vilib>:"CTRE_Phoenix_MotorControl_Set.vi"("error in (no error)"=w451, "Output"=0.0, "Control Mode"=w455, "PhoenixMotorControlDevRef"=w450) -> ()  [unwired: 6 in, 2 out]
                n142 = call <vilib>:"CTRE_Phoenix_MotorControl_Set.vi"("error in (no error)"=w453, "Output"=0.0, "Control Mode"=w457, "PhoenixMotorControlDevRef"=w452) -> ()  [unwired: 6 in, 2 out]
                n143 = call <vilib>:"CTRE_Phoenix_MotorControl_Set.vi"("error in (no error)"=w462, "Output"=0.0, "Control Mode"=w459, "PhoenixMotorControlDevRef"=w463) -> ()  [unwired: 6 in, 2 out]
                n144 = call <vilib>:"CTRE_Phoenix_MotorControl_Set.vi"("error in (no error)"=w464, "Output"=0.0, "Control Mode"=w461, "PhoenixMotorControlDevRef"=w465) -> ()  [unwired: 6 in, 2 out]
                n145 = Wait (ms)(milliseconds to wait=u32 100) -> ()  [unwired: 1 out]
              }
            }
          }
        }
      }
    }
    frame "RIGHT" {
      n146 = while {
        shift-right: [w491] -> _
        shift-left: w477 -> [w490]
        shift-right: [w489] -> _
        shift-left: w478 -> [w488]
        tunnel: w476 -> [w486]
        tunnel: w475 -> [w485]
        tunnel: w474 -> [w484]
        tunnel: w473 -> [w483]
        tunnel: w472 -> [w482]
        tunnel: w471 -> [w481]
        tunnel: w470 -> [w480]
        tunnel: w469 -> [w479]
        stop <- w487 stop-if-true
        n147 = case shown="\"R\", Default" w490 {
          selector: w490 -> [w504 w616]
          tunnel: [w492 w617] -> w491
          tunnel: [w493 w613] -> w489
          tunnel: w488 -> [w503 w615]
          tunnel: [w494 w614] -> w487
          tunnel: w486 -> [w501 w612]
          tunnel: w485 -> [w502 w611]
          tunnel: w484 -> [w499 w610]
          tunnel: w483 -> [w500 w609]
          tunnel: w482 -> [w498 w608]
          tunnel: w481 -> [w497 w607]
          tunnel: w480 -> [w496 w606]
          tunnel: w479 -> [w495 w605]
          frame "L" {
            n148 = case shown="\"2\"" w503 {
              tunnel: w504 -> [w573 w576 w602]
              tunnel: [w573 w576 w602] -> w492
              tunnel: [w571 "5" ("t") "5" ("t")] -> w493
              tunnel: [FALSE FALSE TRUE] -> w494
              tunnel: w501 -> [w520 _ w601]
              tunnel: w502 -> [w519 _ w600]
              tunnel: w500 -> [w516 _ w599]
              tunnel: w498 -> [w513 _ w590]
              tunnel: w497 -> [w511 _ w589]
              tunnel: w496 -> [w508 _ w588]
              tunnel: w495 -> [w509 _ w587]
              tunnel: w499 -> [w505 _ w585]
              frame "1", Default {
                w543 = T9 7 items=["PercentOutput"=0, "Position"=1, "Velocity"=2, "Current"=3, "Follower"=5, "MotionProfile"=6, "MotionMagic"=7, "MotionMagicArc"=8, "MotionProfileArc"=10, "Disabled"=15] ("Control Mode")
                w544 = T9 7 items=["PercentOutput"=0, "Position"=1, "Velocity"=2, "Current"=3, "Follower"=5, "MotionProfile"=6, "MotionMagic"=7, "MotionMagicArc"=8, "MotionProfileArc"=10, "Disabled"=15] ("Control Mode")
                w569 = T9 7 items=["PercentOutput"=0, "Position"=1, "Velocity"=2, "Current"=3, "Follower"=5, "MotionProfile"=6, "MotionMagic"=7, "MotionMagicArc"=8, "MotionProfileArc"=10, "Disabled"=15] ("Control Mode")
                w570 = T9 7 items=["PercentOutput"=0, "Position"=1, "Velocity"=2, "Current"=3, "Follower"=5, "MotionProfile"=6, "MotionMagic"=7, "MotionMagicArc"=8, "MotionProfileArc"=10, "Disabled"=15] ("Control Mode")
                n149 = call <vilib>:"CTRE_Phoenix_MotorControl_SetSelectedSensorPosition.vi"("error in (no error)"=w508, "New Sensor Position"=0, "PhoenixMotorControlDevRef"=w509) -> ("error out"=w506:errorcluster, "PhoenixMotorControlDevRef"=w507:T2)  [unwired: 7 in]
                n150 = call <vilib>:"CTRE_Phoenix_MotorControl_SetSelectedSensorPosition.vi"("error in (no error)"=w513, "New Sensor Position"=0, "PhoenixMotorControlDevRef"=w511) -> ("error out"=w512:errorcluster, "PhoenixMotorControlDevRef"=w510:T2)  [unwired: 7 in]
                n151 = call <vilib>:"CTRE_Phoenix_MotorControl_SetSelectedSensorPosition.vi"("error in (no error)"=w519, "New Sensor Position"=0, "PhoenixMotorControlDevRef"=w520) -> ("error out"=w517:errorcluster, "PhoenixMotorControlDevRef"=w518:T2)  [unwired: 7 in]
                n152 = call <vilib>:"CTRE_Phoenix_MotorControl_SetSelectedSensorPosition.vi"("error in (no error)"=w516, "New Sensor Position"=0, "PhoenixMotorControlDevRef"=w505) -> ("error out"=w514:errorcluster, "PhoenixMotorControlDevRef"=w515:T2)  [unwired: 7 in]
                n153 = call <vilib>:"CTRE_Phoenix_MotorControl_ConfigAllowableClosedLoopError.vi"("error in (no error)"=w514, "slotIdx"=u32 0, "allowableClosedLoopError"=200, "PhoenixMotorControlDevRef"=w515) -> ("error out"=w549:errorcluster, "PhoenixMotorControlDevRef"=w550:T2)  [unwired: 6 in]
                n154 = call <vilib>:"CTRE_Phoenix_MotorControl_ConfigAllowableClosedLoopError.vi"("error in (no error)"=w506, "slotIdx"=u32 0, "allowableClosedLoopError"=200, "PhoenixMotorControlDevRef"=w507) -> ("error out"=w532:errorcluster, "PhoenixMotorControlDevRef"=w533:T2)  [unwired: 6 in]
                n155 = call <vilib>:"CTRE_Phoenix_MotorControl_ConfigAllowableClosedLoopError.vi"("error in (no error)"=w517, "slotIdx"=u32 0, "allowableClosedLoopError"=200, "PhoenixMotorControlDevRef"=w518) -> ("error out"=w553:errorcluster, "PhoenixMotorControlDevRef"=w554:T2)  [unwired: 6 in]
                n156 = call <vilib>:"CTRE_Phoenix_MotorControl_ConfigAllowableClosedLoopError.vi"("error in (no error)"=w512, "slotIdx"=u32 0, "allowableClosedLoopError"=200, "PhoenixMotorControlDevRef"=w510) -> ("error out"=w530:errorcluster, "PhoenixMotorControlDevRef"=w531:T2)  [unwired: 6 in]
                n157 = Wait (ms)(milliseconds to wait=u32 4500) -> ()  [unwired: 1 out]
                n158 = call <vilib>:"CTRE_Phoenix_MotorControl_Set.vi"("error in (no error)"=w532, "Output"=40000.0, "Control Mode"=w543, "PhoenixMotorControlDevRef"=w533) -> ("error out"=w539:errorcluster, "PhoenixMotorControlDevRef"=w540:T2)  [unwired: 6 in]
                n159 = call <vilib>:"CTRE_Phoenix_MotorControl_Set.vi"("error in (no error)"=w530, "Output"=40000.0, "Control Mode"=w544, "PhoenixMotorControlDevRef"=w531) -> ("error out"=w537:errorcluster, "PhoenixMotorControlDevRef"=w538:T2)  [unwired: 6 in]
                n160 = call <vilib>:"CTRE_Phoenix_MotorControl_Set.vi"("error in (no error)"=w549, "Output"=40000.0, "Control Mode"=w569, "PhoenixMotorControlDevRef"=w550) -> ("error out"=w557:errorcluster, "PhoenixMotorControlDevRef"=w558:T2)  [unwired: 6 in]
                n161 = call <vilib>:"CTRE_Phoenix_MotorControl_Set.vi"("error in (no error)"=w553, "Output"=40000.0, "Control Mode"=w570, "PhoenixMotorControlDevRef"=w554) -> ("error out"=w555:errorcluster, "PhoenixMotorControlDevRef"=w556:T2)  [unwired: 6 in]
                n162 = call-poly <vilib>:"CTRE_Phoenix_MotorController_Get_Enhanced.vi"("PhoenixMotorControlDevRef"=w540, "error in"=w539) -> ("Closed-loop Error"=→"Closed-loop Error RF 13":i32)  [unwired: 8 in, 5 out]
                n163 = call-poly <vilib>:"CTRE_Phoenix_MotorController_Get_Enhanced.vi"("PhoenixMotorControlDevRef"=w538, "error in"=w537) -> ("Closed-loop Error"=→"Closed-loop Error LR 13":i32)  [unwired: 8 in, 5 out]
                n164 = call-poly <vilib>:"CTRE_Phoenix_MotorController_Get_Enhanced.vi"("PhoenixMotorControlDevRef"=w558, "error in"=w557) -> ("Closed-loop Error"=w568:i32)  [unwired: 8 in, 5 out]
                "Closed-loop Error RF 14" <- w568
                n165 = call-poly <vilib>:"CTRE_Phoenix_MotorController_Get_Enhanced.vi"("PhoenixMotorControlDevRef"=w556, "error in"=w555) -> ("Closed-loop Error"=w567:i32)  [unwired: 8 in, 5 out]
                "Closed-loop Error LR 14" <- w567
                n166 = Absolute Value(x=w568) -> (abs(x)=w564:i32)
                n167 = Absolute Value(x=w567) -> (abs(x)=w563:i32)
                n168 = Add(x=w564, y=w563) -> (x+y=w566:i32)
                n169 = Divide(x=w566, y=2) -> (x/y=w562:dbl)
                n170 = Greater?(x=w562, y=300.0) -> (0:w546:bool)
                n171 = Select(t="1", s=w546, f="2") -> (s? t:f=w571:string)
              }
              frame "2" {
                n172 = while {
                  stop <- w578 stop-if-true
                  n173 = call <vilib>:"Get_YPRHfH.vi"() -> ("YRPHfH"=w581:T10)  [unwired: 11 in]
                  n174 = Unbundle By Name(w581) -> ("Yaw"=w580:dbl)
                  "Yaw 3" <- w580
                  n175 = call-poly <vilib>:"PID.vi"("output range"=cluster{"output high":dbl, "output low":dbl} {"output high"=0.25, "output low"=-0.25}, "PID gains"="PID gains 3", "process variable"=w580, "setpoint"="setpoint 3") -> ()  [unwired: 6 in, 2 out]
                  n176 = Less?(x=w580, y=-89.0) -> (x < y?=w578:bool)
                }
                n177 = Wait (ms)(milliseconds to wait=u32 1500) -> ()  [unwired: 1 out]
              }
              frame "5" {
                (unwired) 0 ("New Sensor Position")
                (unwired) 0 ("New Sensor Position")
                w592 = T9 0 items=["PercentOutput"=0, "Position"=1, "Velocity"=2, "Current"=3, "Follower"=5, "MotionProfile"=6, "MotionMagic"=7, "MotionMagicArc"=8, "MotionProfileArc"=10, "Disabled"=15] ("Control Mode")
                w594 = T9 0 items=["PercentOutput"=0, "Position"=1, "Velocity"=2, "Current"=3, "Follower"=5, "MotionProfile"=6, "MotionMagic"=7, "MotionMagicArc"=8, "MotionProfileArc"=10, "Disabled"=15] ("Control Mode")
                (unwired) 0 ("New Sensor Position")
                (unwired) 0 ("New Sensor Position")
                w596 = T9 0 items=["PercentOutput"=0, "Position"=1, "Velocity"=2, "Current"=3, "Follower"=5, "MotionProfile"=6, "MotionMagic"=7, "MotionMagicArc"=8, "MotionProfileArc"=10, "Disabled"=15] ("Control Mode")
                w598 = T9 0 items=["PercentOutput"=0, "Position"=1, "Velocity"=2, "Current"=3, "Follower"=5, "MotionProfile"=6, "MotionMagic"=7, "MotionMagicArc"=8, "MotionProfileArc"=10, "Disabled"=15] ("Control Mode")
                n178 = call <vilib>:"CTRE_Phoenix_MotorControl_Set.vi"("error in (no error)"=w600, "Output"=0.0, "Control Mode"=w598, "PhoenixMotorControlDevRef"=w601) -> ()  [unwired: 6 in, 2 out]
                n179 = call <vilib>:"CTRE_Phoenix_MotorControl_Set.vi"("error in (no error)"=w599, "Output"=0.0, "Control Mode"=w596, "PhoenixMotorControlDevRef"=w585) -> ()  [unwired: 6 in, 2 out]
                n180 = call <vilib>:"CTRE_Phoenix_MotorControl_Set.vi"("error in (no error)"=w590, "Output"=0.0, "Control Mode"=w594, "PhoenixMotorControlDevRef"=w589) -> ()  [unwired: 6 in, 2 out]
                n181 = call <vilib>:"CTRE_Phoenix_MotorControl_Set.vi"("error in (no error)"=w588, "Output"=0.0, "Control Mode"=w592, "PhoenixMotorControlDevRef"=w587) -> ()  [unwired: 6 in, 2 out]
                n182 = Wait (ms)(milliseconds to wait=u32 100) -> ()  [unwired: 1 out]
              }
            }
          }
          frame "R", Default {
            n183 = case shown="\"2\"" w615 {
              tunnel: w616 -> [w686 w689 w715]
              tunnel: [w686 w689 w715] -> w617
              tunnel: [w684 "5" ("t") "5" ("t")] -> w613
              tunnel: [FALSE FALSE TRUE] -> w614
              tunnel: w612 -> [w633 _ w714]
              tunnel: w611 -> [w632 _ w713]
              tunnel: w610 -> [w628 _ w712]
              tunnel: w609 -> [w629 _ w711]
              tunnel: w608 -> [w625 _ w702]
              tunnel: w607 -> [w623 _ w701]
              tunnel: w606 -> [w620 _ w700]
              tunnel: w605 -> [w621 _ w699]
              frame "1", Default {
                w656 = T9 7 items=["PercentOutput"=0, "Position"=1, "Velocity"=2, "Current"=3, "Follower"=5, "MotionProfile"=6, "MotionMagic"=7, "MotionMagicArc"=8, "MotionProfileArc"=10, "Disabled"=15] ("Control Mode")
                w657 = T9 7 items=["PercentOutput"=0, "Position"=1, "Velocity"=2, "Current"=3, "Follower"=5, "MotionProfile"=6, "MotionMagic"=7, "MotionMagicArc"=8, "MotionProfileArc"=10, "Disabled"=15] ("Control Mode")
                w682 = T9 7 items=["PercentOutput"=0, "Position"=1, "Velocity"=2, "Current"=3, "Follower"=5, "MotionProfile"=6, "MotionMagic"=7, "MotionMagicArc"=8, "MotionProfileArc"=10, "Disabled"=15] ("Control Mode")
                w683 = T9 7 items=["PercentOutput"=0, "Position"=1, "Velocity"=2, "Current"=3, "Follower"=5, "MotionProfile"=6, "MotionMagic"=7, "MotionMagicArc"=8, "MotionProfileArc"=10, "Disabled"=15] ("Control Mode")
                n184 = call <vilib>:"CTRE_Phoenix_MotorControl_SetSelectedSensorPosition.vi"("error in (no error)"=w620, "New Sensor Position"=0, "PhoenixMotorControlDevRef"=w621) -> ("error out"=w618:errorcluster, "PhoenixMotorControlDevRef"=w619:T2)  [unwired: 7 in]
                n185 = call <vilib>:"CTRE_Phoenix_MotorControl_SetSelectedSensorPosition.vi"("error in (no error)"=w625, "New Sensor Position"=0, "PhoenixMotorControlDevRef"=w623) -> ("error out"=w624:errorcluster, "PhoenixMotorControlDevRef"=w622:T2)  [unwired: 7 in]
                n186 = call <vilib>:"CTRE_Phoenix_MotorControl_SetSelectedSensorPosition.vi"("error in (no error)"=w632, "New Sensor Position"=0, "PhoenixMotorControlDevRef"=w633) -> ("error out"=w630:errorcluster, "PhoenixMotorControlDevRef"=w631:T2)  [unwired: 7 in]
                n187 = call <vilib>:"CTRE_Phoenix_MotorControl_SetSelectedSensorPosition.vi"("error in (no error)"=w629, "New Sensor Position"=0, "PhoenixMotorControlDevRef"=w628) -> ("error out"=w626:errorcluster, "PhoenixMotorControlDevRef"=w627:T2)  [unwired: 7 in]
                n188 = call <vilib>:"CTRE_Phoenix_MotorControl_ConfigAllowableClosedLoopError.vi"("error in (no error)"=w626, "slotIdx"=u32 0, "allowableClosedLoopError"=200, "PhoenixMotorControlDevRef"=w627) -> ("error out"=w662:errorcluster, "PhoenixMotorControlDevRef"=w663:T2)  [unwired: 6 in]
                n189 = call <vilib>:"CTRE_Phoenix_MotorControl_ConfigAllowableClosedLoopError.vi"("error in (no error)"=w618, "slotIdx"=u32 0, "allowableClosedLoopError"=200, "PhoenixMotorControlDevRef"=w619) -> ("error out"=w645:errorcluster, "PhoenixMotorControlDevRef"=w646:T2)  [unwired: 6 in]
                n190 = call <vilib>:"CTRE_Phoenix_MotorControl_ConfigAllowableClosedLoopError.vi"("error in (no error)"=w630, "slotIdx"=u32 0, "allowableClosedLoopError"=200, "PhoenixMotorControlDevRef"=w631) -> ("error out"=w666:errorcluster, "PhoenixMotorControlDevRef"=w667:T2)  [unwired: 6 in]
                n191 = call <vilib>:"CTRE_Phoenix_MotorControl_ConfigAllowableClosedLoopError.vi"("error in (no error)"=w624, "slotIdx"=u32 0, "allowableClosedLoopError"=200, "PhoenixMotorControlDevRef"=w622) -> ("error out"=w643:errorcluster, "PhoenixMotorControlDevRef"=w644:T2)  [unwired: 6 in]
                n192 = Wait (ms)(milliseconds to wait=u32 4000) -> ()  [unwired: 1 out]
                n193 = call <vilib>:"CTRE_Phoenix_MotorControl_Set.vi"("error in (no error)"=w645, "Output"=35655.0, "Control Mode"=w656, "PhoenixMotorControlDevRef"=w646) -> ("error out"=w652:errorcluster, "PhoenixMotorControlDevRef"=w653:T2)  [unwired: 6 in]
                n194 = call <vilib>:"CTRE_Phoenix_MotorControl_Set.vi"("error in (no error)"=w643, "Output"=35655.0, "Control Mode"=w657, "PhoenixMotorControlDevRef"=w644) -> ("error out"=w650:errorcluster, "PhoenixMotorControlDevRef"=w651:T2)  [unwired: 6 in]
                n195 = call <vilib>:"CTRE_Phoenix_MotorControl_Set.vi"("error in (no error)"=w662, "Output"=35655.0, "Control Mode"=w682, "PhoenixMotorControlDevRef"=w663) -> ("error out"=w670:errorcluster, "PhoenixMotorControlDevRef"=w671:T2)  [unwired: 6 in]
                n196 = call <vilib>:"CTRE_Phoenix_MotorControl_Set.vi"("error in (no error)"=w666, "Output"=35655.0, "Control Mode"=w683, "PhoenixMotorControlDevRef"=w667) -> ("error out"=w668:errorcluster, "PhoenixMotorControlDevRef"=w669:T2)  [unwired: 6 in]
                n197 = call-poly <vilib>:"CTRE_Phoenix_MotorController_Get_Enhanced.vi"("PhoenixMotorControlDevRef"=w653, "error in"=w652) -> ("Closed-loop Error"=→"Closed-loop Error RF 11":i32)  [unwired: 8 in, 5 out]
                n198 = call-poly <vilib>:"CTRE_Phoenix_MotorController_Get_Enhanced.vi"("PhoenixMotorControlDevRef"=w651, "error in"=w650) -> ("Closed-loop Error"=→"Closed-loop Error LR 11":i32)  [unwired: 8 in, 5 out]
                n199 = call-poly <vilib>:"CTRE_Phoenix_MotorController_Get_Enhanced.vi"("PhoenixMotorControlDevRef"=w671, "error in"=w670) -> ("Closed-loop Error"=w681:i32)  [unwired: 8 in, 5 out]
                "Closed-loop Error RF 12" <- w681
                n200 = call-poly <vilib>:"CTRE_Phoenix_MotorController_Get_Enhanced.vi"("PhoenixMotorControlDevRef"=w669, "error in"=w668) -> ("Closed-loop Error"=w680:i32)  [unwired: 8 in, 5 out]
                "Closed-loop Error LR 12" <- w680
                n201 = Absolute Value(x=w681) -> (abs(x)=w677:i32)
                n202 = Absolute Value(x=w680) -> (abs(x)=w676:i32)
                n203 = Add(x=w677, y=w676) -> (x+y=w679:i32)
                n204 = Divide(x=w679, y=2) -> (x/y=w675:dbl)
                n205 = Greater?(x=w675, y=200.0) -> (0:w659:bool)
                n206 = Select(t="1", s=w659, f="2") -> (s? t:f=w684:string)
              }
              frame "2" {
                n207 = while {
                  stop <- w691 stop-if-true
                  n208 = call <vilib>:"Get_YPRHfH.vi"() -> ("YRPHfH"=w694:T10)  [unwired: 11 in]
                  n209 = Unbundle By Name(w694) -> ("Yaw"=w693:dbl)
                  "Yaw 2" <- w693
                  n210 = call-poly <vilib>:"PID.vi"("output range"=cluster{"output high":dbl, "output low":dbl} {"output high"=0.25, "output low"=-0.25}, "PID gains"="PID gains 2", "process variable"=w693, "setpoint"="setpoint 2") -> ()  [unwired: 6 in, 2 out]
                  n211 = Less?(x=w693, y=-89.0) -> (x < y?=w691:bool)
                }
                n212 = Wait (ms)(milliseconds to wait=u32 1500) -> ()  [unwired: 1 out]
              }
              frame "5" {
                (unwired) 0 ("New Sensor Position")
                (unwired) 0 ("New Sensor Position")
                w704 = T9 0 items=["PercentOutput"=0, "Position"=1, "Velocity"=2, "Current"=3, "Follower"=5, "MotionProfile"=6, "MotionMagic"=7, "MotionMagicArc"=8, "MotionProfileArc"=10, "Disabled"=15] ("Control Mode")
                w706 = T9 0 items=["PercentOutput"=0, "Position"=1, "Velocity"=2, "Current"=3, "Follower"=5, "MotionProfile"=6, "MotionMagic"=7, "MotionMagicArc"=8, "MotionProfileArc"=10, "Disabled"=15] ("Control Mode")
                (unwired) 0 ("New Sensor Position")
                (unwired) 0 ("New Sensor Position")
                w708 = T9 0 items=["PercentOutput"=0, "Position"=1, "Velocity"=2, "Current"=3, "Follower"=5, "MotionProfile"=6, "MotionMagic"=7, "MotionMagicArc"=8, "MotionProfileArc"=10, "Disabled"=15] ("Control Mode")
                w710 = T9 0 items=["PercentOutput"=0, "Position"=1, "Velocity"=2, "Current"=3, "Follower"=5, "MotionProfile"=6, "MotionMagic"=7, "MotionMagicArc"=8, "MotionProfileArc"=10, "Disabled"=15] ("Control Mode")
                n213 = call <vilib>:"CTRE_Phoenix_MotorControl_Set.vi"("error in (no error)"=w713, "Output"=0.0, "Control Mode"=w710, "PhoenixMotorControlDevRef"=w714) -> ()  [unwired: 6 in, 2 out]
                n214 = call <vilib>:"CTRE_Phoenix_MotorControl_Set.vi"("error in (no error)"=w711, "Output"=0.0, "Control Mode"=w708, "PhoenixMotorControlDevRef"=w712) -> ()  [unwired: 6 in, 2 out]
                n215 = call <vilib>:"CTRE_Phoenix_MotorControl_Set.vi"("error in (no error)"=w702, "Output"=0.0, "Control Mode"=w706, "PhoenixMotorControlDevRef"=w701) -> ()  [unwired: 6 in, 2 out]
                n216 = call <vilib>:"CTRE_Phoenix_MotorControl_Set.vi"("error in (no error)"=w700, "Output"=0.0, "Control Mode"=w704, "PhoenixMotorControlDevRef"=w699) -> ()  [unwired: 6 in, 2 out]
                n217 = Wait (ms)(milliseconds to wait=u32 100) -> ()  [unwired: 1 out]
              }
            }
          }
        }
      }
    }
    frame "Alternative 2" {
      w719 = "RobotDrive Motors" ("Name")
      # "This is some simple sample code to drive your robot curving one direction and then the other."
      # "stand still"
      # "other way for 0.5 second"
      # "turn for 1 second"
      n218 = call <vilib>:"WPI_RobotDriveRefNum Registry Get.vi"("refnum name"="Left and Right Motors") -> ("RobotDriveDevRef"=w735:T11)  [unwired: 1 in, 9 out]
      n219 = call-poly <vilib>:"WPI_RobotDriveArcadeDrive.vi"("Y axis value"=0.5 ("X axis value"), "X axis value"=-0.25, "RobotDriveDevRef"=w735) -> ("Motor Values"=w718:dbl[], "RobotDriveDevRef"=w728:T11)  [unwired: 1 in, 6 out]
      n220 = call-poly <vilib>:"NT Write Value.vi"("Numeric Array"=w718, "Name"=w719) -> ()  [unwired: 9 in, 1 out]
      n221 = call <vilib>:"WPI_RobotDriveDelayAndUpdateSafety.vi"("Delay (s)"=1.0, "RobotDriveDevRef"=w728) -> ("RobotDriveDevRef 2"=w729:T11)  [unwired: 8 in, 1 out]
      n222 = call-poly <vilib>:"WPI_RobotDriveArcadeDrive.vi"("Y axis value"=-0.25 ("X axis value"), "X axis value"=0.5, "RobotDriveDevRef"=w729) -> ("Motor Values"=w720:dbl[], "RobotDriveDevRef"=w730:T11)  [unwired: 1 in, 6 out]
      n223 = call-poly <vilib>:"NT Write Value.vi"("Numeric Array"=w720, "Name"=w719) -> ()  [unwired: 9 in, 1 out]
      n224 = call <vilib>:"WPI_RobotDriveDelayAndUpdateSafety.vi"("Delay (s)"=0.5, "RobotDriveDevRef"=w730) -> ("RobotDriveDevRef 2"=w731:T11)  [unwired: 8 in, 1 out]
      n225 = call-poly <vilib>:"WPI_RobotDriveArcadeDrive.vi"("Y axis value"=0.0 ("X axis value"), "X axis value"=0.0, "RobotDriveDevRef"=w731) -> ("Motor Values"=w721:dbl[])  [unwired: 1 in, 7 out]
      n226 = call-poly <vilib>:"NT Write Value.vi"("Numeric Array"=w721, "Name"=w719) -> ()  [unwired: 9 in, 1 out]
    }
    frame "Alternative 1" {
    }
    frame Default {
    }
    frame "Your Turn" {
    }
  }
